vi "fast scanner v1.2.vi"() -> ()   [LabVIEW 2015]
uses:
  libs/Controls/outofrange.ctl
  libs/Controls/loopclock.ctl
  libs/Controls/fast scanner.ctl
  <vilib>/Utility/file.llb/Write Delimited Spreadsheet (DBL).vi
  <vilib>/Utility/file.llb/Write Delimited Spreadsheet (I64).vi
  Zaber A Series/Zaber A Series.lvlib
panel:
  out "DPP Configuration":T1={"reset_recovery_time"=300, "edge_peaking_time"=5, "flat_top"=5, "peaking_time"=25, "gain"=1.0, "max_risetime"=35.0, "fast_filter_thr"=100, "zero_peak_freq"=5.0, "inverted_input"=0, "base_offset"=0, "reset_threshold"=1000, "overflow_recovery"=0, "tail_coefficient"=0.0, "energy_filter_thr"=25, "energy_baseline_thr"=25, "max_peaking_time"=0, "edge_flat_top"=1, "time_constant"=0.0, "baseline_samples"=64, "other_param"=0}
  in  "Data folder path":path=path "d:/Users/XRF/Desktop/Scan DATA"
  out "DANTE loaded":bool
  out "IP added":bool
  out "Library Initialized":bool
  out "DANTE configured":bool
  out "Enum":T2=enum."MoveToStartPoint"
  out "scan mode":bool
  out "Port":refnum<visa-resource-name>
  out "MotorsReady":bool
  out "Speed 2":T3 scale=0.0..30.0
  in  "Tab Control":T4(tab)
  in  "StopMotion":bool
  in  "GoToZ":bool
  in  "GoToY":bool
  in  "GoToX":bool
  in  "GoTo Z [mm]":dbl format="%#.8g"
  in  "GoTo Y [mm]":dbl format="%#.8g"
  in  "GoTo X [mm]":dbl format="%#.8g"
  in  "Reduced Speed":bool
  in  "Speed Z [mm/s]":dbl(slide) caption="Z Speed\n[mm/s]" min=0.5 max=10.0 step=0.5 scale=0.5..10.0
  in  "XY Speed\n[mm/s]":dbl(slide)=1.0 min=1.0 max=75.0 step=1.0 scale=1.0..75.0
  in  "Away":bool
  in  "Closer":bool
  in  "Right":bool
  in  "Left":bool
  in  "Down":bool
  in  "Up":bool
  out "X [mm]":dbl format="%#.8g"
  out "Y [mm]":dbl format="%#.8g"
  out "Z [mm]":dbl format="%#.3g"
  out "Assignment":cluster{"Microstep Size":dbl, "Device":string}[](array[cluster])
  in  "Acceleration [mm/s^2]":dbl=1.0 min=1.0 max=488.0
  out "SpectraPlot":dbl[](graph) caption="Waveform Graph"
  in  "APPEARANCE_CursorVis":bool
  in  "APPEARANCE_Log/Lin":bool=TRUE
  out "stats out":T5
  out "identifier out":string
  in  "IP Address":string="10.96.0.110"
  out "Progress":u32 caption="%" min=1 step=1
  in  "Preset Time [s]":dbl=1.0 min=0.2 step=0.1
  out "Elapsed Time":dbl caption="Elapsed Time [s]" format="%#_4g"
  in  "MEASUREMENT_Start":bool
  in  "INIT DANTE":bool
  in  "Close DANTE":bool
  out "ROI Begin":u32 caption="ROI begin channel"
  out "ROI End":u32 caption="ROI end channel"
  in  "Config. file path":path=path "Configuration files/DefaultParameters.xml"
  in  "And dist [mm]":dbl=1.0 caption="Single line measurement time:" min=0.0 step=0.1
  in  "X velocity [mm/s]":dbl=50.0 min=0.0 step=0.1
  out "Total scan time [s]":dbl=1.0 min=0.0 step=0.1
  out "Total line time [s]":dbl=1.0 min=0.0 step=0.1
  out "Acq time [s]":dbl=1.0 min=0.0 step=0.1
  in  "AcqStartDelay":dbl caption="Acq start delay [ms]"
  in  "Abort scan":bool
  out "Acc time [s]":dbl=1.0 min=0.0 step=0.1
  out "Acc dist [mm]":dbl=1.0 caption="Single line measurement time:" min=0.0 step=0.1
  in  "X accel":dbl caption="X acceleration [mm/s^2]"
  out "Line #":i32=1 caption="/" min=0 step=1
  out "X scan velocity [mm/s]":dbl=1.0 min=0.0 step=0.1
  in  "QUICKSCAN_Start":bool
  out "Y error":T6
  out "X error":T6
  out "total # of points":i32=1 min=0 step=1
  out "Y steps":i32=1 min=1 step=1
  out "X steps":i32=1 min=1 step=1
  in  "step Y [mm]":dbl=1.0 min=0.0 step=0.1
  in  "Y end [mm]":dbl=1.0
  in  "Y start [mm]":dbl
  in  "step X [mm]":dbl=1.0 min=0.0 step=0.1
  in  "X end [mm]":dbl=1.0
  in  "X start [mm]":dbl
  in  "PresetVal":u32 caption="Time per pixel [ms]"
  out "X speed error":T6
  out "total line #":i32=1 caption="/" min=0 step=1
  out "Return movement time [s]":dbl=1.0 min=0.0 step=0.1
  out "ROI map":u32[][](graph)
  out "Sum spectra per line":u32[](graph)
  out "Spectra":u16[][](graph)
  out "scan timing [ms]":dbl[][](array[numeric])
  out "Y positions array":dbl[](array[numeric])
  out "X start position":dbl
  out "X end position":dbl
  in  "Precision [mm]":dbl=0.1
  out "ZaberError":errorcluster
  out "Loop Speed [1/s]":dbl caption="Elapsed Time [s]" format="%#_2f"
  # "waiting \ntill stage \nreaches \nproper speed"
  # "sending \nmovement \ncommand"
  # "waiting till \nstage stops \n(breaking)"
  # "aquisition"
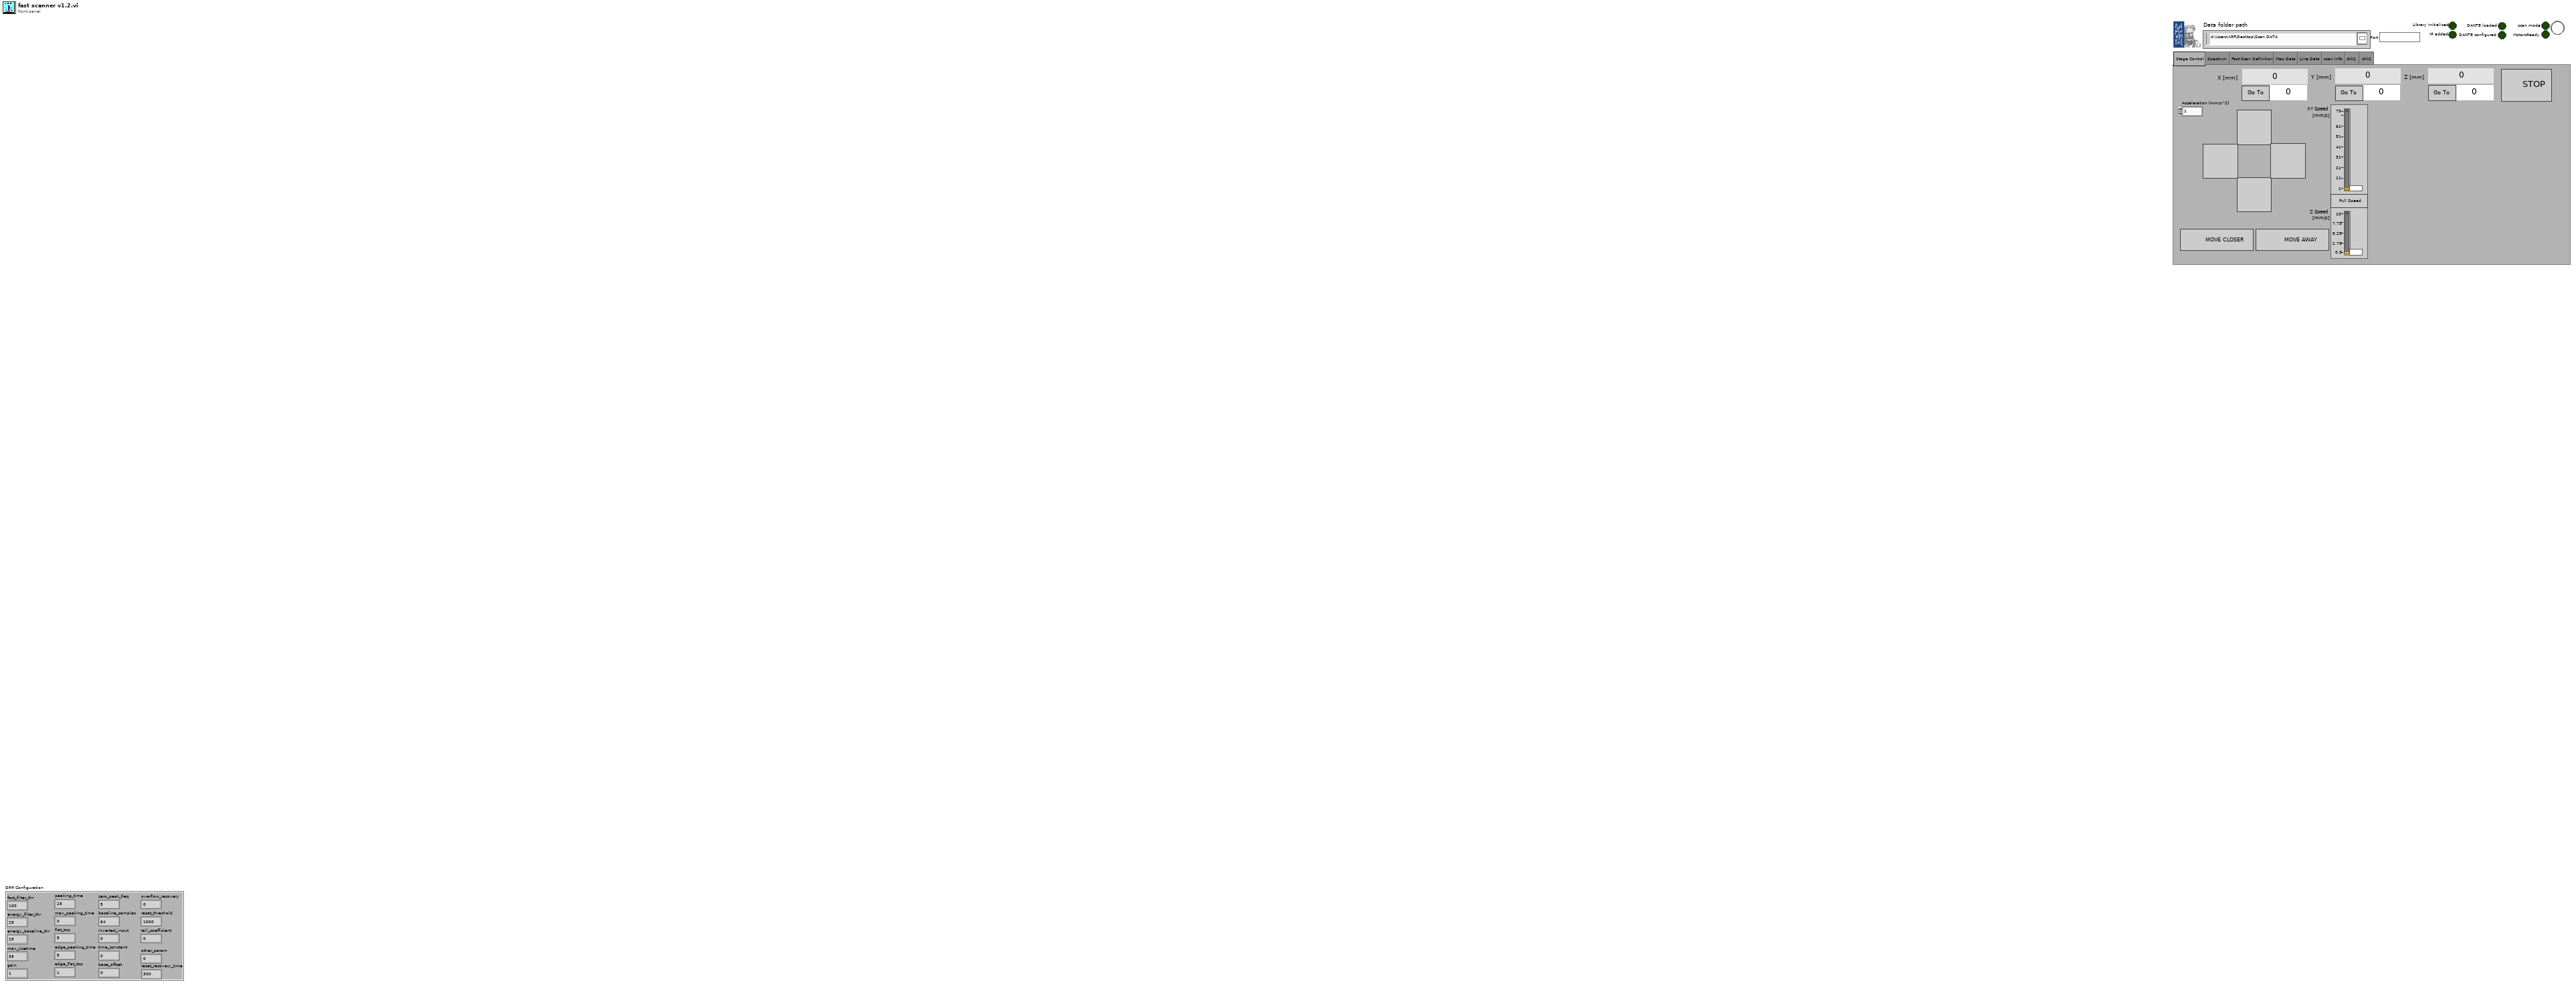
[diagram p1: front panel]
types:
  T1 = cluster{"reset_recovery_time":u32, "edge_peaking_time":u32, "flat_top":u32, "peaking_time":u32, "gain":dbl, "max_risetime":dbl, "fast_filter_thr":u32, "zero_peak_freq":dbl, "inverted_input":u8, "base_offset":u32, "reset_threshold":u32, "overflow_recovery":u32, "tail_coefficient":dbl, "energy_filter_thr":u32, "energy_baseline_thr":u32, "max_peaking_time":u32, "edge_flat_top":u32, "time_constant":dbl, "baseline_samples":u32, "other_param":u32}
  T2 = typedef "fast scanner.ctl" = enum16{"Initialisation", "IDLE", "Acquire", "PrepareMap", "MoveToStartPoint", "AcquireLine", "Close"}
  T3 = typedef "loopclock.ctl" = dbl
  T4 = enum32{"Stage Control", "Spectrum", "Fast Scan Definition", "Map Data", "Line Data", "scan info", "chk1", "chk2"}
  T5 = cluster{u64, u64, dbl, dbl, u32, u32, u32, u32, u32, u32, u32, u32, u32, u32, u32}
  T6 = typedef "outofrange.ctl" = bool
  T7 = cluster{"X min":dbl, "X max":dbl, "Y min":dbl, "Y max":dbl, "Z min":dbl, "Z max":dbl}
  T8 = enum32{"Size Tabs To Contents", "Size All Tabs to Largest Tab", "Fixed Tab Size"}
  T9 = enum8{"Enabled", "Disabled", "Disabled and Grayed Out"}
  T10 = typedef "ConfigurationDPP.ctl" = cluster{"reset_recovery_time":u32, "edge_peaking_time":u32, "flat_top":u32, "peaking_time":u32, "gain":dbl, "max_risetime":dbl, "fast_filter_thr":u32, "zero_peak_freq":dbl, "inverted_input":u8, "base_offset":u32, "reset_threshold":u32, "overflow_recovery":u32, "tail_coefficient":dbl, "energy_filter_thr":u32, "energy_baseline_thr":u32, "max_peaking_time":u32, "edge_flat_top":u32, "time_constant":dbl, "baseline_samples":u32, "other_param":u32}
  T11 = typedef "LVMinMaxIncTypeDef.ctl" = cluster{"Minimum":dbl, "Maximum":dbl, "Increment":dbl}
  T12 = typedef "LVRangeTypeDef.ctl" = cluster{"Minimum":dbl, "Maximum":dbl, "Increment":dbl, "Minor Increment":dbl, "Start":dbl}
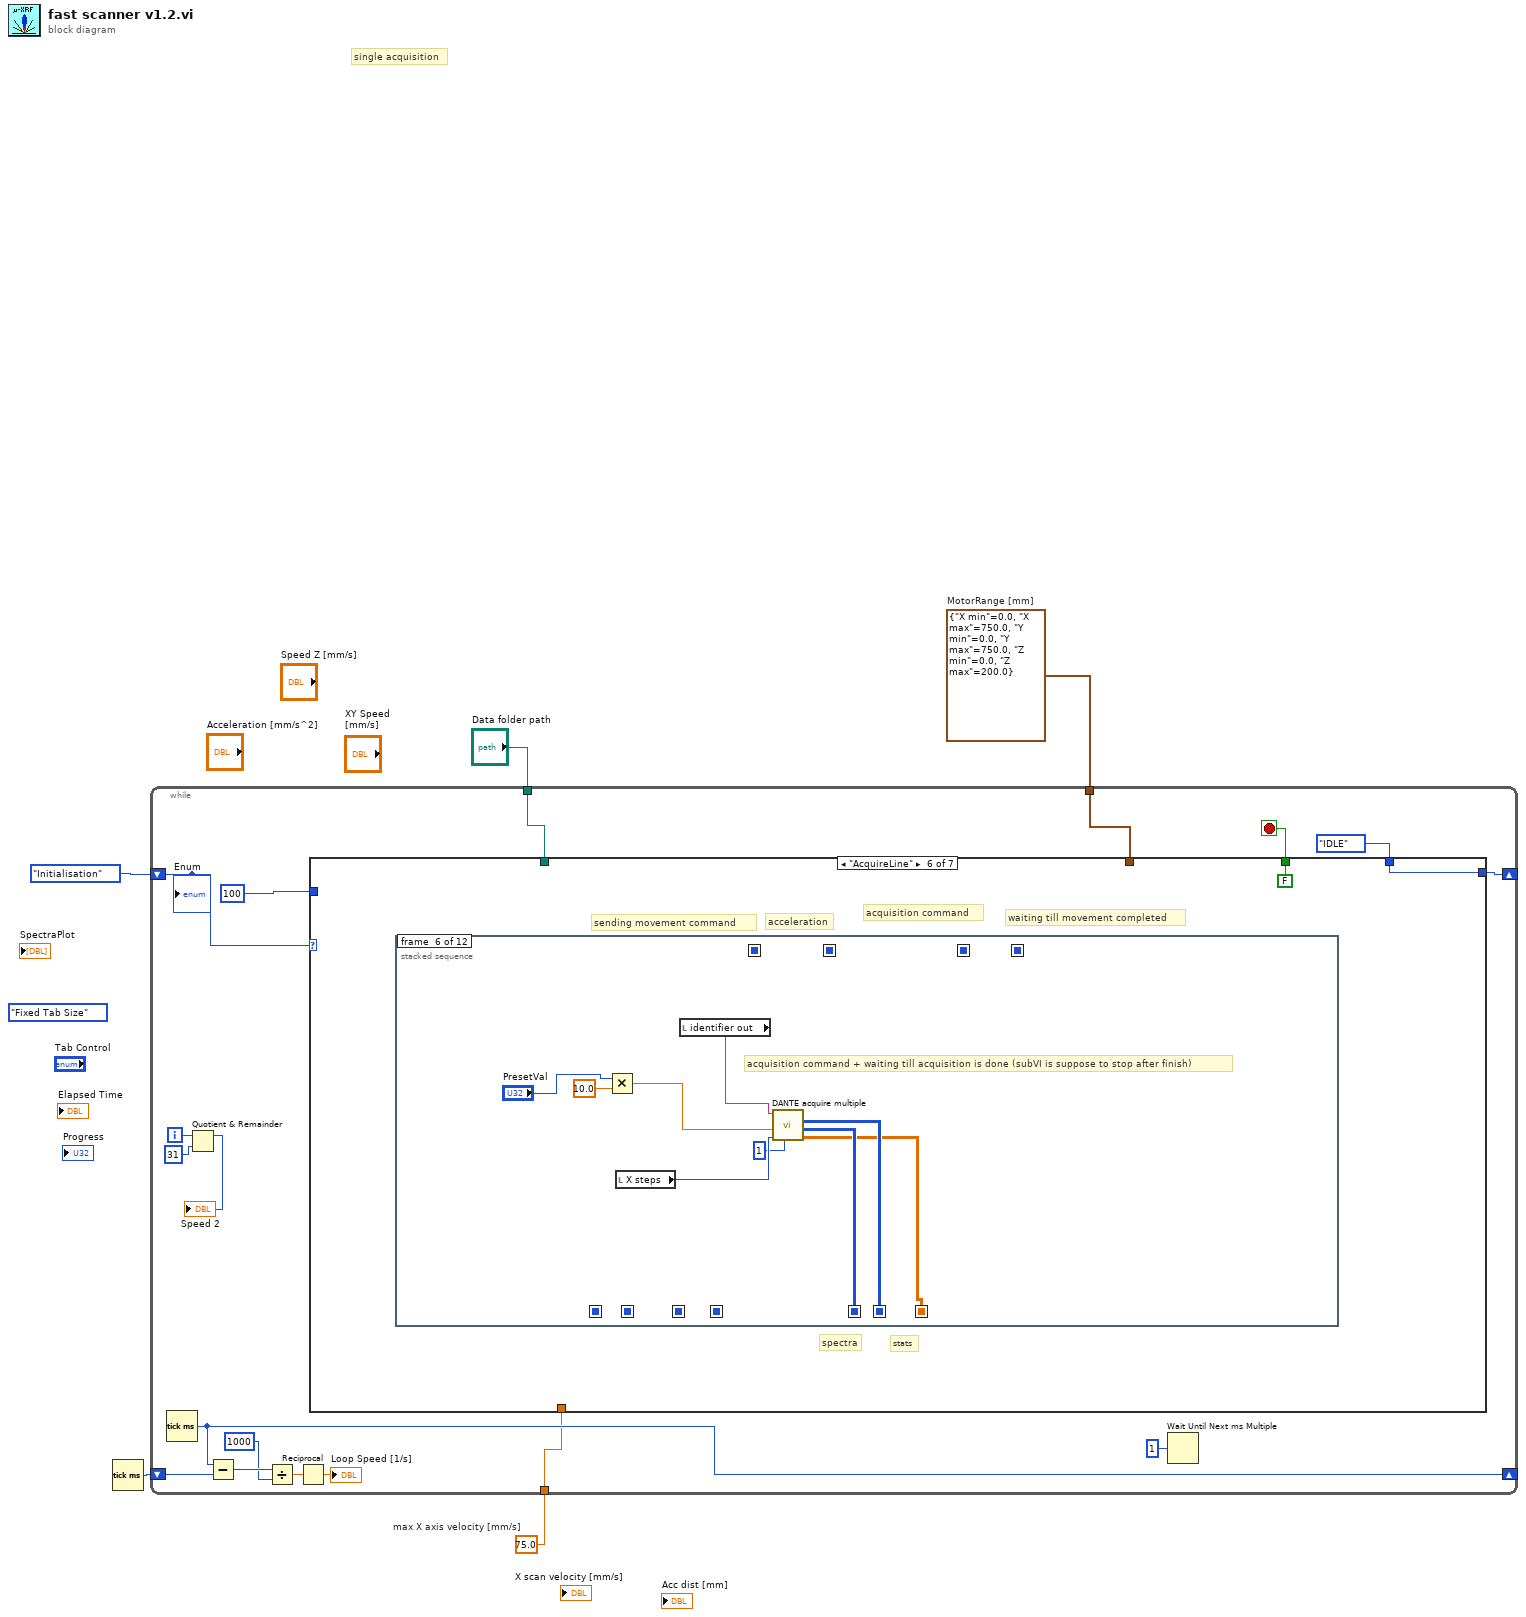
[diagram p0: block diagram]
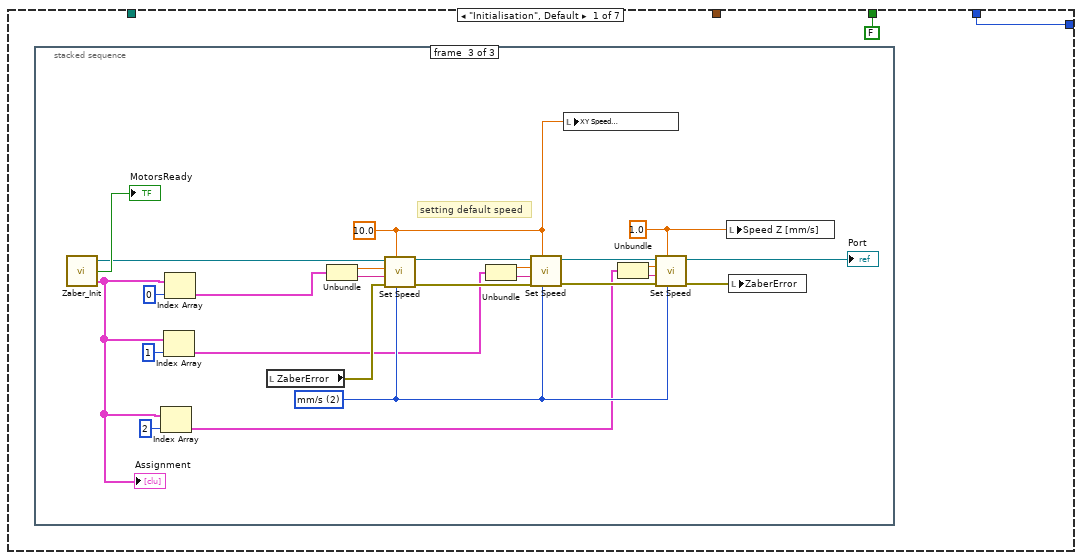
[diagram p2: hidden frame]
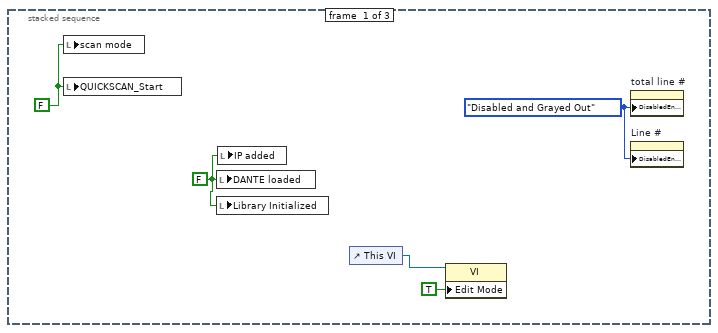
[diagram p3: hidden frame]
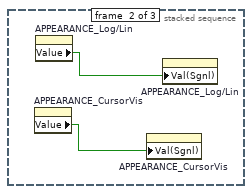
[diagram p4: hidden frame]
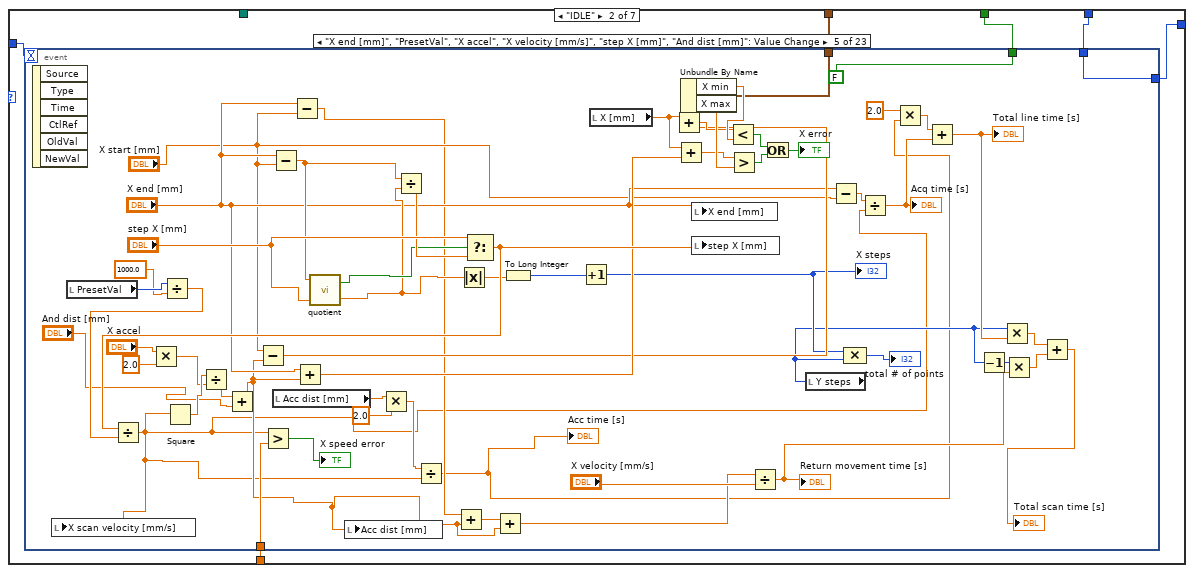
[diagram p5: hidden frame]
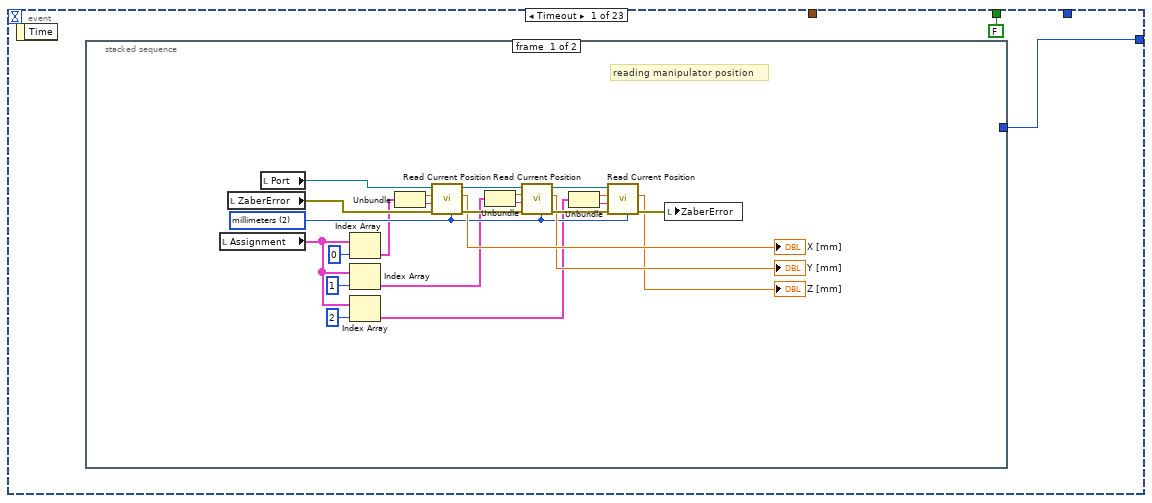
[diagram p6: hidden frame]
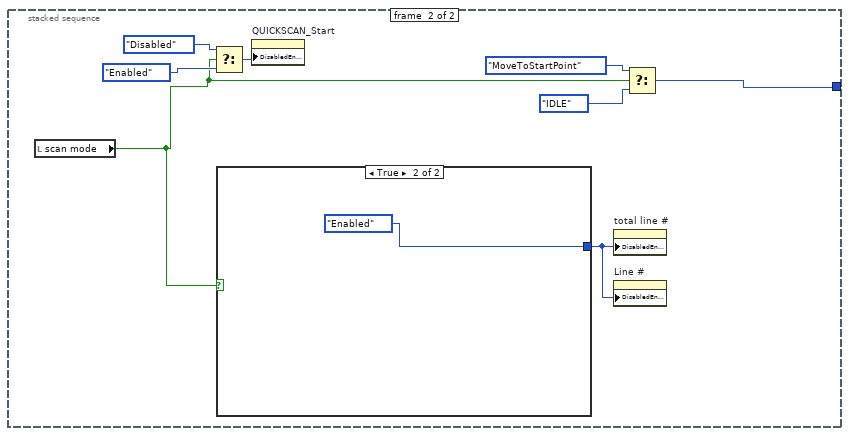
[diagram p7: hidden frame]
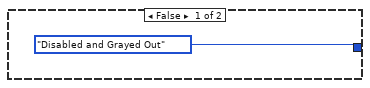
[diagram p8: hidden frame]
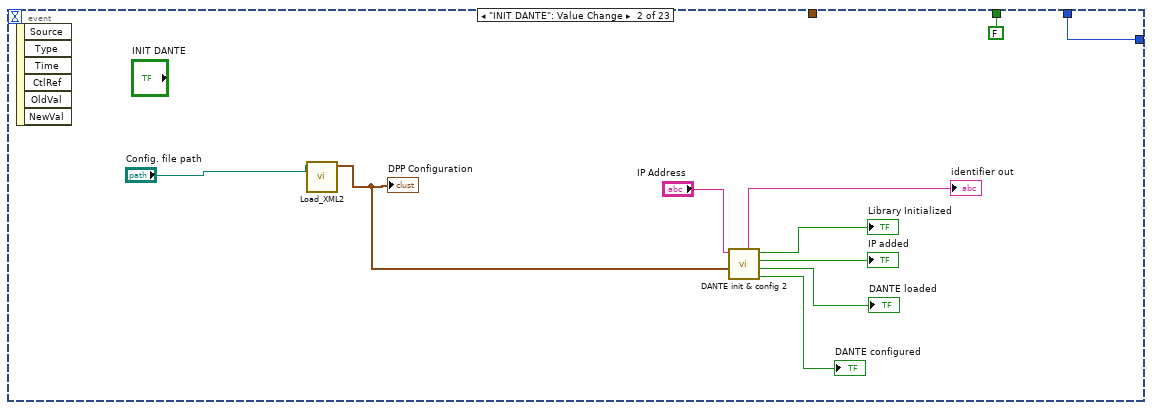
[diagram p9: hidden frame]
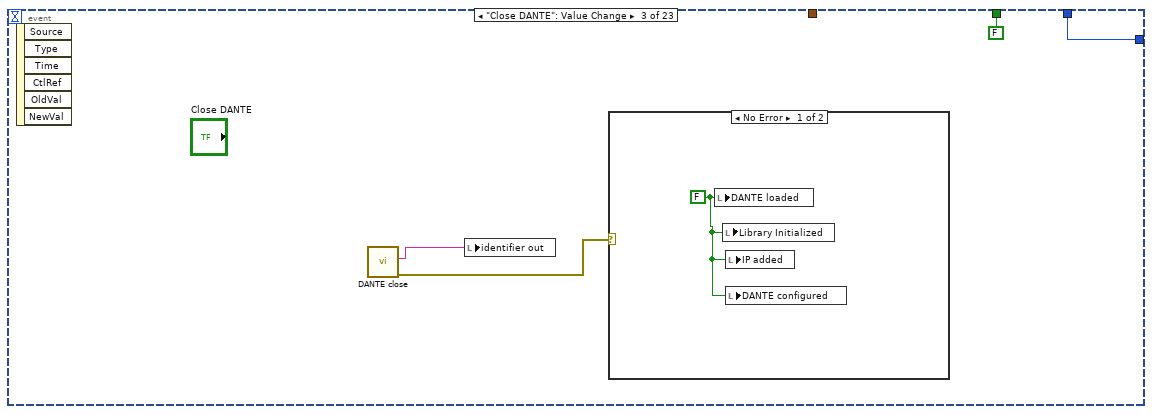
[diagram p10: hidden frame]
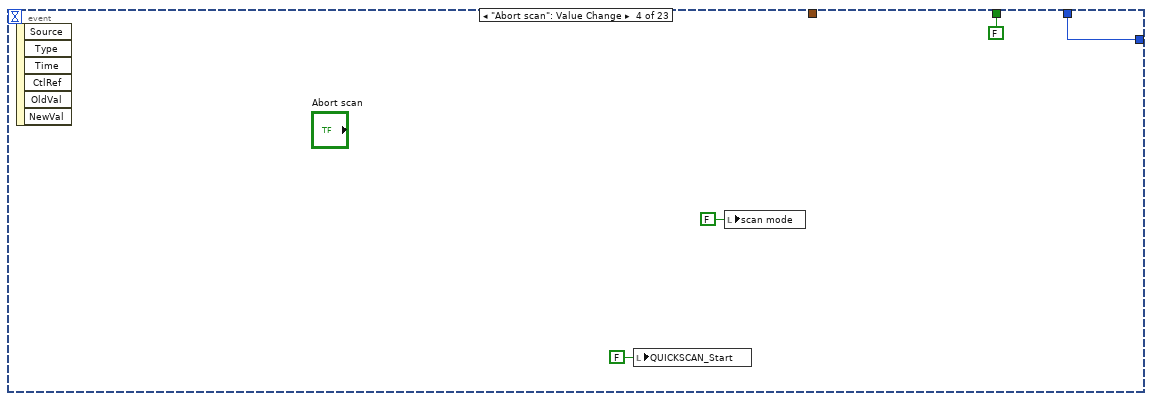
[diagram p12: hidden frame]
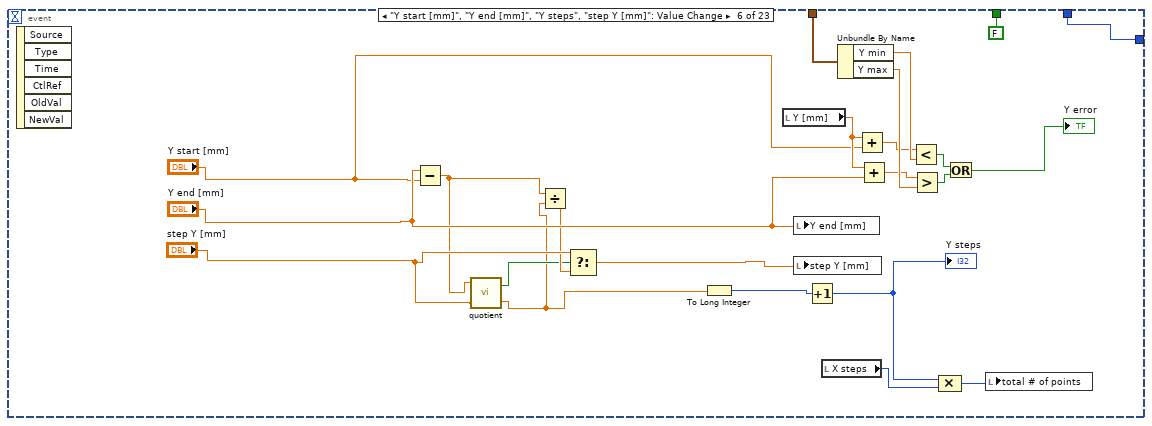
[diagram p13: hidden frame]
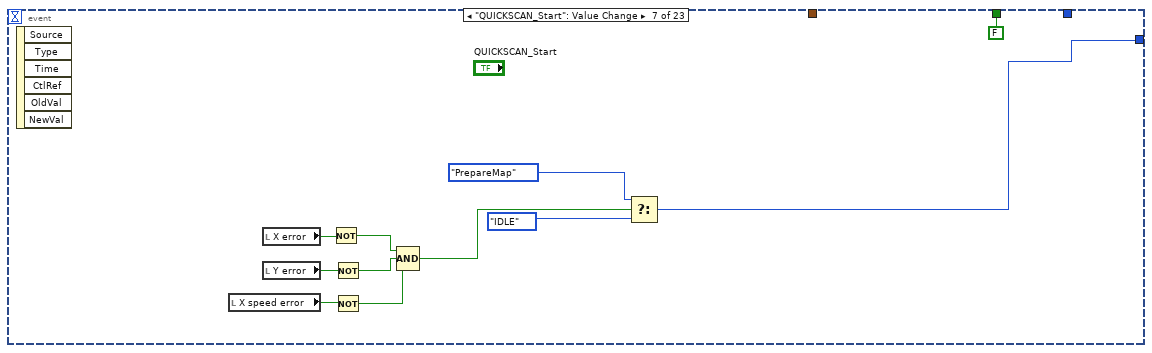
[diagram p14: hidden frame]
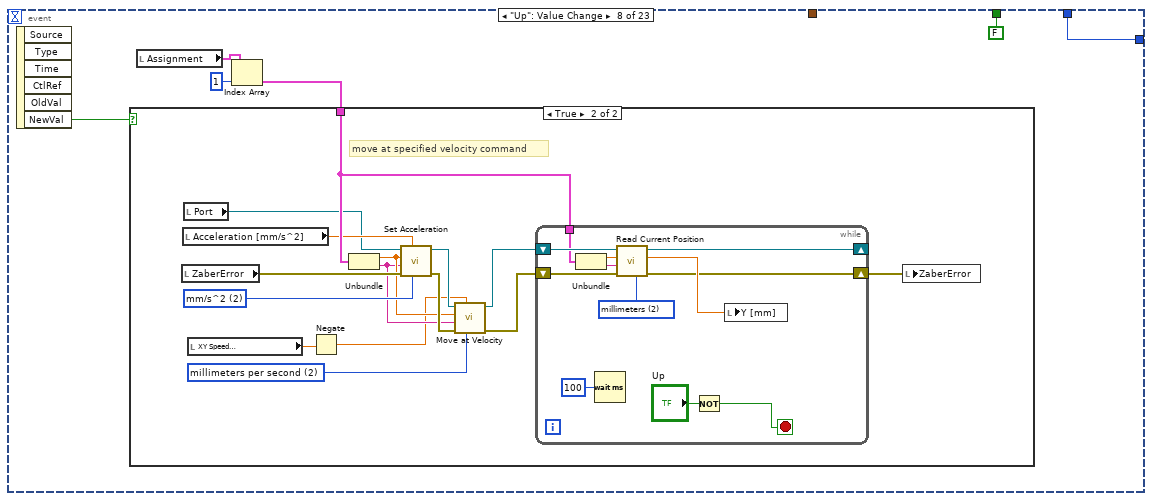
[diagram p15: hidden frame]
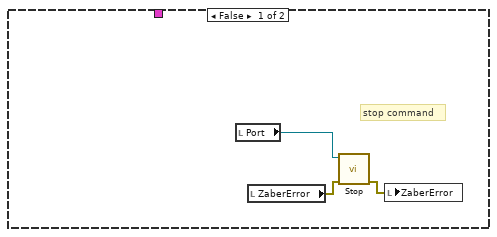
[diagram p16: hidden frame]
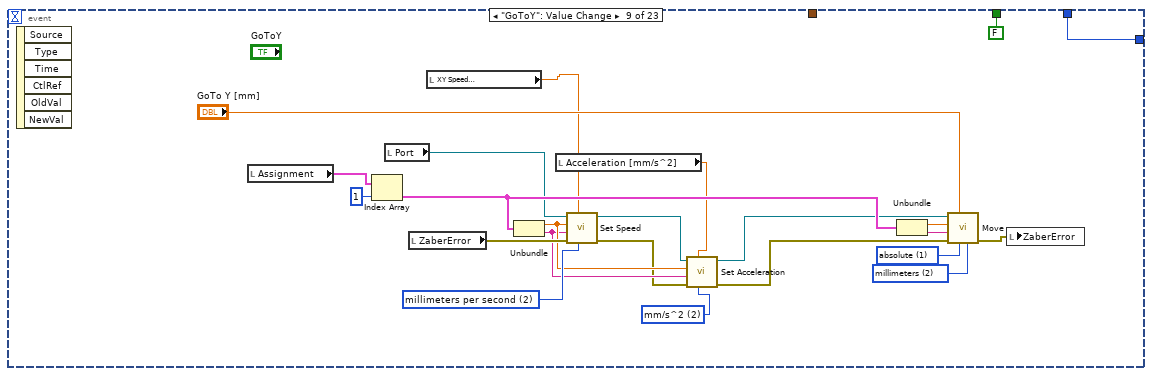
[diagram p17: hidden frame]
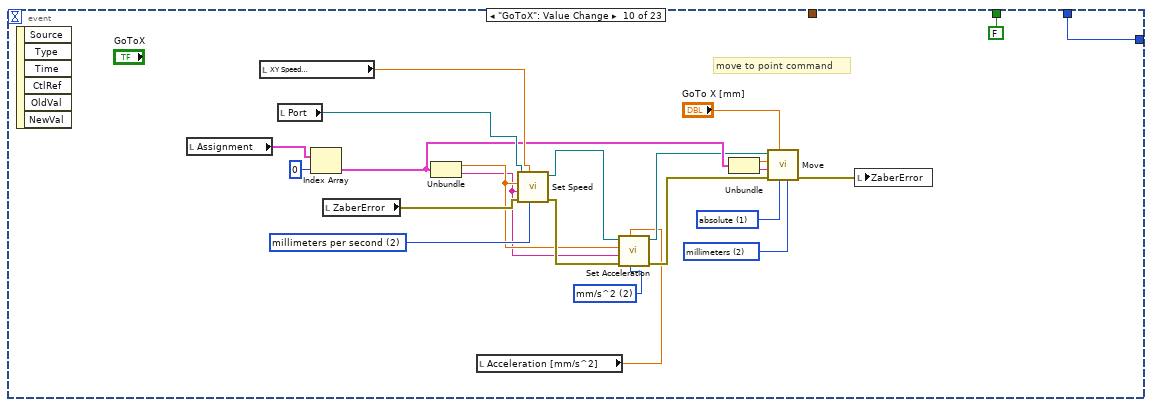
[diagram p18: hidden frame]
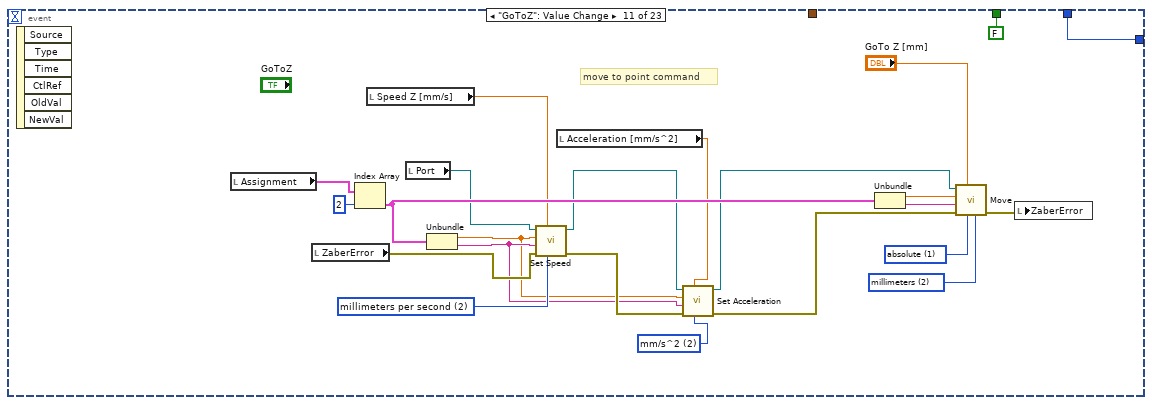
[diagram p19: hidden frame]
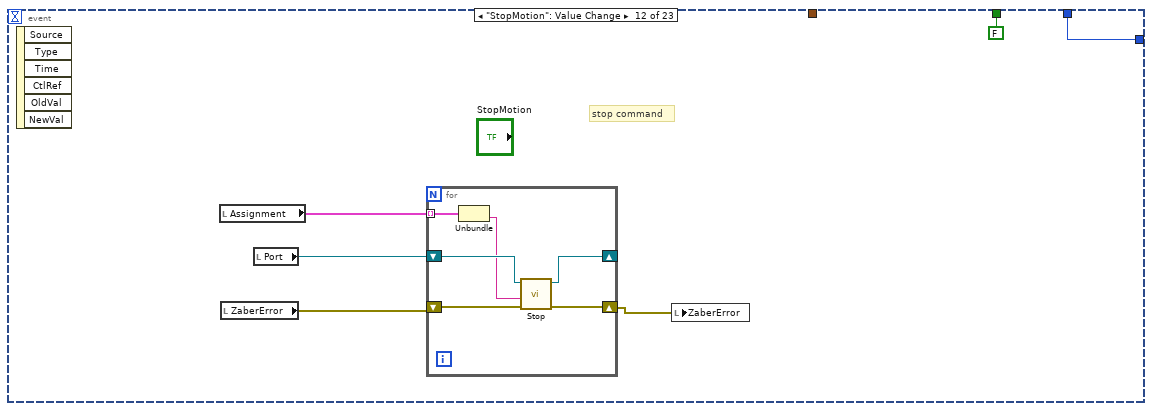
[diagram p20: hidden frame]
diagram:
  w2 = 75.0  # max X axis velocity [mm/s]
  w4 = T7 {"X min"=0.0, "X max"=750.0, "Y min"=0.0, "Y max"=750.0, "Z min"=0.0, "Z max"=200.0}  # MotorRange [mm]
  (unwired) T8."Fixed Tab Size" ("Tab Size")
  # "single acquisition"
  n1 = Tick Count (ms)() -> (millisecond timer value=w5:u32)
  n2 = while {
    shift-right: [w12] -> _
    shift-left: fast_scanner."Initialisation" ("Enum") -> [w8]
    shift-right: [w19] -> _
    shift-left: w5 -> [w23]
    tunnel: w4 -> [w9]
    tunnel: w2 -> [w7]
    tunnel: "Data folder path" -> [w6]
    i -> [w18]
    stop <- w11 stop-if-true
    n3 = Tick Count (ms)() -> (millisecond timer value=w19:u32)
    n4 = Quotient & Remainder(x=w18, y=31) -> (x-y*floor(x/y)=→"Speed 2":i32)  [unwired: 1 out]
    n5 = Subtract(x=w19, y=w23) -> (x-y=w21:u32)
    n6 = Divide(x=w21, y=u32 1000) -> (x/y=w22:dbl)
    n7 = Reciprocal(x=w22) -> (1/x=→"Loop Speed [1/s]":dbl)
    n8 = case shown="\"AcquireLine\"" w8 {
      tunnel: 100 ("LoopTimer [ms]") -> [_ w59 _ _ _ _ _]
      tunnel: [w25 w61 fast_scanner."IDLE" ("Enum") w582 fast_scanner."AcquireLine" ("Enum") w692 fast_scanner."Close" ("Enum")] -> w12
      tunnel: [FALSE ("VI stop") w60 FALSE ("VI stop") FALSE ("VI stop") FALSE ("VI stop") FALSE ("VI stop") TRUE ("VI stop")] -> w11
      tunnel: fast_scanner."IDLE" ("Enum") -> [w25 w63 _ w582 _ w692 _]
      tunnel: w9 -> [_ w62 _ _ _ _ _]
      tunnel: w7 -> [_ w58 _ _ _ _ _]
      tunnel: w6 -> [_ _ _ _ _ _ _]
      frame "Initialisation", Default {
        n9 = stacked-sequence {
          frame #0 {
            w26 = FALSE ("DANTE loaded")
            w27 = T9."Disabled and Grayed Out" ("Disabled")
            w28 = FALSE ("batch mode")
            n10 = local write "scan mode"(w28) -> ()
            n11 = local write "QUICKSCAN_Start"(w28) -> ()
            n12 = local write "DANTE loaded"(w26) -> ()
            n13 = local write "Library Initialized"(w26) -> ()
            n14 = local write "IP added"(w26) -> ()
            n15 = control-ref of="This VI"() -> (w29:refnum<vi>)
            n16 = property class="VI"(reference=w29, "Edit Mode"=TRUE ("Edit Mode On Open")) -> ()  [unwired: 1 in, 2 out]
            n17 = property on="total line #" class="DigNum (strict)"("DisabledEnum"=w27) -> ()  [unwired: 2 in, 2 out]
            n18 = property on="Line #" class="DigNum (strict)"("DisabledEnum"=w27) -> ()  [unwired: 2 in, 2 out]
          }
          frame #1 {
            n19 = property on="APPEARANCE_CursorVis" class="Bool (strict)"() -> ("Value"=w31:bool)  [unwired: 2 in, 2 out]
            n20 = property on="APPEARANCE_Log/Lin" class="Bool (strict)"() -> ("Value"=w32:bool)  [unwired: 2 in, 2 out]
            n21 = property on="APPEARANCE_CursorVis" class="Bool (strict)"("Val(Sgnl)"=w31) -> ()  [unwired: 2 in, 2 out]
            n22 = property on="APPEARANCE_Log/Lin" class="Bool (strict)"("Val(Sgnl)"=w32) -> ()  [unwired: 2 in, 2 out]
          }
          frame #2 {
            w42 = 1.0 ("New Speed")
            w43 = 10.0 ("New Speed")
            w46 = u16 2 items=["device units", "microns/s", "mm/s", "inches/s", "degrees/s"] ("Units (0: data)")
            # "setting default speed"
            n23 = call "Zaber_Init.vi"() -> ("Assignment"=w47:cluster{"Microstep Size":dbl, "Device":string}[], "Axes Ass"=→"MotorsReady":bool, "VISA resource name out"=w55:refnum<visa-resource-name>)
            "Assignment" <- w47
            n24 = Index Array(array=w47, index=2) -> (element=w34:cluster{"Microstep Size":dbl, "Device":string})
            n25 = Index Array(array=w47, index=1) -> (element=w36:cluster{"Microstep Size":dbl, "Device":string})
            n26 = Index Array(array=w47, index=0) -> (element=w41:cluster{"Microstep Size":dbl, "Device":string})
            n27 = local read "ZaberError"() -> (w56:errorcluster)
            n28 = Unbundle(w41) -> ("Microstep Size"=w40:dbl, "Device"=w39:string)
            n29 = call "Set Speed.vi"("Units (0: data)"=w46, "New Speed"=w43, "error in (no error)"=w56, "Device and Axis"=w39, "Microstep Size (0)"=w40, "VISA resource name"=w55) -> ("error out"=w52:errorcluster, "VISA resource name out"=w51:refnum<visa-resource-name>)  [unwired: 4 in]
            n30 = Unbundle(w36) -> ("Microstep Size"=w37:dbl, "Device"=w38:string)
            n31 = call "Set Speed.vi"("Units (0: data)"=w46, "New Speed"=w43, "error in (no error)"=w52, "Device and Axis"=w38, "Microstep Size (0)"=w37, "VISA resource name"=w51) -> ("error out"=w49:errorcluster, "VISA resource name out"=w50:refnum<visa-resource-name>)  [unwired: 4 in]
            n32 = local write "XY Speed\n[mm/s]"(w43) -> ()
            n33 = Unbundle(w34) -> ("Microstep Size"=w35:dbl, "Device"=w33:string)
            n34 = call "Set Speed.vi"("Units (0: data)"=w46, "New Speed"=w42, "error in (no error)"=w49, "Device and Axis"=w33, "Microstep Size (0)"=w35, "VISA resource name"=w50) -> ("error out"=w45:errorcluster, "VISA resource name out"=→"Port":refnum<visa-resource-name>)  [unwired: 4 in]
            n35 = local write "Speed Z [mm/s]"(w42) -> ()
            n36 = local write "ZaberError"(w45) -> ()
          }
        }
      }
      frame "IDLE" {
        n37 = event shown="[4] \"X end [mm]\", \"PresetVal\", \"X accel\", \"X velocity [mm/s]\", \"step X [mm]\", \"And dist [mm]\": Value Change" {
          selector: _ -> [_ _ _ _ _ _ _ _ _ _ _ _ _ _ _ _ _ _ _ _ _ _ _]
          dyn-events: _ -> [_ _ _ _ _ _ _ _ _ _ _ _ _ _ _ _ _ _ _ _ _ _ _]
          timeout: w59 -> [_ _ _ _ _ _ _ _ _ _ _ _ _ _ _ _ _ _ _ _ _ _ _]
          tunnel: [FALSE ("VI stop") FALSE ("VI stop") FALSE ("VI stop") FALSE ("VI stop") FALSE ("VI stop") FALSE ("VI stop") FALSE ("VI stop") FALSE ("VI stop") FALSE ("VI stop") FALSE ("VI stop") FALSE ("VI stop") FALSE ("VI stop") FALSE ("VI stop") FALSE ("VI stop") FALSE ("VI stop") FALSE ("VI stop") FALSE ("VI stop") FALSE ("VI stop") TRUE ("VI stop") FALSE ("VI stop") FALSE ("VI stop") FALSE ("VI stop") FALSE ("VI stop")] -> w60
          tunnel: [w64 w109 w113 w117 w175 w196 w199 w213 w267 w290 w313 w320 w331 w366 w401 w437 w472 w516 w533 fast_scanner."Acquire" ("Enum") w551 w556 w560] -> w61
          tunnel: w63 -> [_ w109 w113 w117 w175 w196 _ w213 w267 w290 w313 w320 w331 w366 w401 w437 w472 w516 _ _ w551 w556 w560]
          tunnel: w62 -> [_ _ _ _ w163 w182 _ _ _ _ _ _ _ _ _ _ _ _ _ _ _ _ _]
          tunnel: w58 -> [_ _ _ _ w152 _ _ _ _ _ _ _ _ _ _ _ _ _ _ _ _ _ _]
          event Timeout {
            n38 = event-data() -> ()  [unwired: 1 in, 1 out]
            n39 = stacked-sequence {
              tunnel: [_ w97] -> w64
              frame #0 {
                w76 = u16 2 items=["microsteps", "microns", "millimeters", "inches"] ("Units (0: microsteps)")
                # "reading manipulator position"
                n40 = local read "Assignment"() -> (w75:cluster{"Microstep Size":dbl, "Device":string}[])
                n41 = local read "ZaberError"() -> (w88:errorcluster)
                n42 = local read "Port"() -> (w89:refnum<visa-resource-name>)
                n43 = Index Array(array=w75, index=0) -> (element=w74:cluster{"Microstep Size":dbl, "Device":string})
                n44 = Index Array(array=w75, index=1) -> (element=w70:cluster{"Microstep Size":dbl, "Device":string})
                n45 = Index Array(array=w75, index=2) -> (element=w66:cluster{"Microstep Size":dbl, "Device":string})
                n46 = Unbundle(w74) -> ("Microstep Size"=w73:dbl, "Device"=w72:string)
                n47 = call "Read Current Position.vi"("Units (0: microsteps)"=w76, "error in (no error)"=w88, "Device and Axis"=w72, "Microstep Size (0)"=w73, "VISA resource name"=w89) -> ("error out"=w87:errorcluster, "Position"=→"X [mm]":dbl, "VISA resource name out"=w86:refnum<visa-resource-name>)  [unwired: 4 in]
                n48 = Unbundle(w70) -> ("Microstep Size"=w71:dbl, "Device"=w69:string)
                n49 = call "Read Current Position.vi"("Units (0: microsteps)"=w76, "error in (no error)"=w87, "Device and Axis"=w69, "Microstep Size (0)"=w71, "VISA resource name"=w86) -> ("error out"=w85:errorcluster, "Position"=→"Y [mm]":dbl, "VISA resource name out"=w84:refnum<visa-resource-name>)  [unwired: 4 in]
                n50 = Unbundle(w66) -> ("Microstep Size"=w68:dbl, "Device"=w67:string)
                n51 = call "Read Current Position.vi"("Units (0: microsteps)"=w76, "error in (no error)"=w85, "Device and Axis"=w67, "Microstep Size (0)"=w68, "VISA resource name"=w84) -> ("error out"=w83:errorcluster, "Position"=→"Z [mm]":dbl)  [unwired: 4 in, 1 out]
                n52 = local write "ZaberError"(w83) -> ()
              }
              frame #1 {
                n53 = local read "scan mode"() -> (w90:bool)
                n54 = Select(t=T9."Disabled" ("Disabled"), s=w90, f=T9."Enabled" ("Disabled")) -> (s? t:f=w94:T9)
                n55 = case shown="True" w90 {
                  tunnel: [T9."Disabled and Grayed Out" ("Disabled") T9."Enabled" ("Disabled")] -> w91
                  frame False {
                  }
                  frame True {
                  }
                }
                n56 = property on="QUICKSCAN_Start" class="Bool (strict)"("DisabledEnum"=w94) -> ()  [unwired: 2 in, 2 out]
                n57 = property on="total line #" class="DigNum (strict)"("DisabledEnum"=w91) -> ()  [unwired: 2 in, 2 out]
                n58 = property on="Line #" class="DigNum (strict)"("DisabledEnum"=w91) -> ()  [unwired: 2 in, 2 out]
                n59 = Select(t=fast_scanner."MoveToStartPoint" ("Enum"), s=w90, f=fast_scanner."IDLE" ("Enum")) -> (s? t:f=w97:T2)
              }
            }
          }
          event "INIT DANTE": Value Change {
            n60 = event-data() -> ()  [unwired: 1 in, 6 out]
            n61 = call "Load_XML2.vi"("XML File Path 2"="Config. file path") -> ("DPP Configuration"=w100:T10)  [unwired: 10 in]
            "DPP Configuration" <- w100
            n62 = call "DANTE init & config 2.vi"("DPP Configuration"=w100, "IP Address"="IP Address") -> ("DANTE configured"=→"DANTE configured":bool, "DANTE loaded"=→"DANTE loaded":bool, "IP added"=→"IP added":bool, "Library Initialized"=→"Library Initialized":bool, "identifier out"=→"identifier out":string)  [unwired: 5 in]
          }
          event "Close DANTE": Value Change {
            n63 = event-data() -> ()  [unwired: 1 in, 6 out]
            n64 = call "DANTE close.vi"() -> ("error out"=w110:errorcluster, "identifier out"=w111:string)  [unwired: 9 in, 1 out]
            n65 = local write "identifier out"(w111) -> ()
            n66 = case shown="No Error" w110 {
              frame No Error {
                w114 = FALSE ("DANTE loaded")
                n67 = local write "DANTE loaded"(w114) -> ()
                n68 = local write "Library Initialized"(w114) -> ()
                n69 = local write "IP added"(w114) -> ()
                n70 = local write "DANTE configured"(w114) -> ()
              }
              frame Error {
              }
            }
          }
          event "Abort scan": Value Change {
            n71 = event-data() -> ()  [unwired: 1 in, 6 out]
            n72 = local write "QUICKSCAN_Start"(FALSE ("QUICKSCAN_Start")) -> ()
            n73 = local write "scan mode"(FALSE ("scan mode")) -> ()
          }
          event "X end [mm]", "PresetVal", "X accel", "X velocity [mm/s]", "step X [mm]", "And dist [mm]": Value Change {
            n74 = event-data() -> ()  [unwired: 1 in, 6 out]
            n75 = local read "PresetVal"() -> (w159:u32)
            n76 = Multiply(x="X accel", y=2.0) -> (x*y=w154:dbl)
            n77 = Divide(x=w159, y=1000.0 ("x")) -> (x/y=w157:dbl)
            n78 = Subtract(x="X end [mm]", y="X start [mm]") -> (x-y=w146:dbl)
            n79 = local read "Acc dist [mm]"() -> (w124:dbl)
            n80 = Subtract(x="X end [mm]", y="X start [mm]") -> (x-y=w129:dbl)
            n81 = call "quotient.vi"("Y"="step X [mm]", "X"=w146) -> ("s? t:f"=w144:dbl, "x = y?"=w145:bool)  [unwired: 1 in]
            n82 = Multiply(x=w124, y=2.0) -> (x*y=w122:dbl)
            n83 = Divide(x=w146, y=w144) -> (x/y=w148:dbl)
            n84 = Absolute Value(x=w144) -> (abs(x)=w147:dbl)
            n85 = Select(t="step X [mm]", s=w145, f=w148) -> (s? t:f=w161:dbl)
            n86 = Divide(x=w161, y=w157) -> (x/y=w120:dbl)
            n87 = local write "X scan velocity [mm/s]"(w120) -> ()
            n88 = Square(x=w120) -> (x^2=w156:dbl)
            n89 = Divide(x=w156, y=w154) -> (x/y=w126:dbl)
            n90 = Add(x=w126, y="And dist [mm]") -> (x+y=w125:dbl)
            n91 = Subtract(x="X start [mm]", y=w125) -> (x-y=w150:dbl)
            n92 = Greater?(x=w120, y=w152) -> (0:→"X speed error":bool)
            n93 = Add(x="X end [mm]", y=w125) -> (x+y=w151:dbl)
            n94 = local write "Acc dist [mm]"(w125) -> ()
            n95 = Divide(x=w122, y=w120) -> (x/y=w119:dbl)
            "Acc time [s]" <- w119
            n96 = Add(x=w129, y=w125) -> (x+y=w128:dbl)
            n97 = Add(x=w128, y=w125) -> (x+y=w127:dbl)
            n98 = To Long Integer(number=w147) -> (32bit integer=w167:i32)
            n99 = Increment(x=w167) -> (x+1=w143:i32)
            "X steps" <- w143
            n100 = local read "X [mm]"() -> (w171:dbl)
            n101 = Add(x=w171, y=w150) -> (x+y=w166:dbl)
            n102 = Add(x=w171, y=w151) -> (x+y=w165:dbl)
            n103 = Unbundle By Name(w163) -> ("X min"=w172:dbl, "X max"=w170:dbl)
            n104 = local write "X end [mm]"("X end [mm]") -> ()
            n105 = local write "step X [mm]"(w161) -> ()
            n106 = Less?(x=w166, y=w172) -> (x < y?=w168:bool)
            n107 = Greater?(x=w165, y=w170) -> (0:w169:bool)
            n108 = Divide(x=w127, y="X velocity [mm/s]") -> (x/y=w135:dbl)
            "Return movement time [s]" <- w135
            n109 = Or(x=w168, y=w169) -> (x .or. y?=→"X error":bool)
            n110 = local read "Y steps"() -> (w136:i32)
            n111 = Subtract(x="X end [mm]", y="X start [mm]") -> (x-y=w142:dbl)
            n112 = Compound Arithmetic op=MULTIPLY(w143, w136) -> (→"total # of points":i32)
            n113 = Divide(x=w142, y=w120) -> (x/y=w141:dbl)
            "Acq time [s]" <- w141
            n114 = Multiply(x=2.0, y=w119) -> (x*y=w140:dbl)
            n115 = Add(x=w140, y=w141) -> (x+y=w138:dbl)
            "Total line time [s]" <- w138
            n116 = Decrement(x=w136) -> (x-1=w137:i32)
            n117 = Multiply(x=w136, y=w138) -> (x*y=w133:dbl)
            n118 = Multiply(x=w137, y=w135) -> (x*y=w134:dbl)
            n119 = Add(x=w133, y=w134) -> (x+y=→"Total scan time [s]":dbl)
          }
          event "Y start [mm]", "Y end [mm]", "Y steps", "step Y [mm]": Value Change {
            n120 = event-data() -> ()  [unwired: 1 in, 6 out]
            n121 = Subtract(x="Y end [mm]", y="Y start [mm]") -> (x-y=w179:dbl)
            n122 = call "quotient.vi"("Y"="step Y [mm]", "X"=w179) -> ("s? t:f"=w177:dbl, "x = y?"=w178:bool)  [unwired: 1 in]
            n123 = Divide(x=w179, y=w177) -> (x/y=w180:dbl)
            n124 = Select(t="step Y [mm]", s=w178, f=w180) -> (s? t:f=w183:dbl)
            n125 = To Long Integer(number=w177) -> (32bit integer=w194:i32)
            n126 = local read "Y [mm]"() -> (w192:dbl)
            n127 = local write "Y end [mm]"("Y end [mm]") -> ()
            n128 = local write "step Y [mm]"(w183) -> ()
            n129 = Increment(x=w194) -> (x+1=w176:i32)
            "Y steps" <- w176
            n130 = local read "X steps"() -> (w193:i32)
            n131 = Unbundle By Name(w182) -> ("Y min"=w188:dbl, "Y max"=w187:dbl)
            n132 = Add(x=w192, y="Y start [mm]") -> (x+y=w185:dbl)
            n133 = Add(x=w192, y="Y end [mm]") -> (x+y=w184:dbl)
            n134 = Less?(x=w185, y=w188) -> (x < y?=w190:bool)
            n135 = Greater?(x=w184, y=w187) -> (0:w191:bool)
            n136 = Compound Arithmetic op=MULTIPLY(w176, w193) -> (w181:i32)
            n137 = Or(x=w190, y=w191) -> (x .or. y?=→"Y error":bool)
            n138 = local write "total # of points"(w181) -> ()
          }
          event "QUICKSCAN_Start": Value Change {
            n139 = event-data() -> ()  [unwired: 1 in, 6 out]
            n140 = local read "X speed error"() -> (w205:T6)
            n141 = local read "X error"() -> (w203:T6)
            n142 = local read "Y error"() -> (w204:T6)
            n143 = Not(x=w203) -> (.not. x?=w206:T6)
            n144 = Not(x=w204) -> (.not. x?=w207:T6)
            n145 = Not(x=w205) -> (.not. x?=w208:T6)
            n146 = Compound Arithmetic op=AND(w206, w207, w208) -> (w202:T6)
            n147 = Select(t=fast_scanner."PrepareMap" ("Enum"), s=w202, f=fast_scanner."IDLE" ("Enum")) -> (s? t:f=w199:T2)
          }
          event "Up": Value Change {
            n148 = event-data() -> ("NewVal"=w215:bool)  [unwired: 1 in, 5 out]
            n149 = local read "Assignment"() -> (w210:cluster{"Microstep Size":dbl, "Device":string}[])
            n150 = Index Array(array=w210, index=1) -> (element=w211:cluster{"Microstep Size":dbl, "Device":string})
            n151 = case shown="True" w215 {
              tunnel: w211 -> [_ w232]
              frame False {
                # "stop command"
                n152 = local read "Port"() -> (w218:refnum<visa-resource-name>)
                n153 = local read "ZaberError"() -> (w217:errorcluster)
                n154 = call "Stop.vi"("error in (no error)"=w217, "VISA resource name"=w218) -> ("error out"=w216:errorcluster)  [unwired: 8 in, 1 out]
                n155 = local write "ZaberError"(w216) -> ()
              }
              frame True {
                w230 = u16 2 items=["device units", "microns/s^2", "mm/s^2", "inches/s^2", "degrees/s^2"] ("Units (0: data)")
                w220 = u16 2 items=["device speed units", "microns per second", "millimeters per second", "inches per second", "degrees per second"] ("Units (0: device speed units)")
                # "move at specified velocity command"
                n156 = local read "ZaberError"() -> (w228:errorcluster)
                n157 = local read "Acceleration [mm/s^2]"() -> (w229:dbl)
                n158 = local read "Port"() -> (w227:refnum<visa-resource-name>)
                n159 = local read "XY Speed\n[mm/s]"() -> (w231:dbl)
                n160 = Negate(x=w231) -> (-x=w219:dbl)
                n161 = Unbundle(w232) -> ("Microstep Size"=w224:dbl, "Device"=w223:string)
                n162 = call "Set Acceleration.vi"("Units (0: data)"=w230, "New Acceleration"=w229, "error in (no error)"=w228, "Device and Axis"=w223, "Microstep Size (0)"=w224, "VISA resource name"=w227) -> ("error out"=w226:errorcluster, "VISA resource name out"=w225:refnum<visa-resource-name>)  [unwired: 4 in]
                n163 = call "Move at Velocity.vi"("Units (0: device speed units)"=w220, "Velocity"=w219, "error in (no error)"=w226, "Device and Axis"=w223, "Microstep Size (0)"=w224, "VISA resource name"=w225) -> ("error out"=w221:errorcluster, "VISA resource name out"=w222:refnum<visa-resource-name>)  [unwired: 4 in]
                n164 = while {
                  shift-right: [w237] -> _
                  shift-left: w222 -> [w240]
                  shift-right: [w238] -> w233
                  shift-left: w221 -> [w239]
                  tunnel: w232 -> [w236]
                  stop <- w243 stop-if-true
                  w242 = u16 2 items=["microsteps", "microns", "millimeters", "inches"] ("Units (0: microsteps)")
                  n165 = Unbundle(w236) -> ("Microstep Size"=w235:dbl, "Device"=w234:string)
                  n166 = Wait (ms)(milliseconds to wait=u32 100) -> ()  [unwired: 1 out]
                  n167 = call "Read Current Position.vi"("Units (0: microsteps)"=w242, "error in (no error)"=w239, "Device and Axis"=w234, "Microstep Size (0)"=w235, "VISA resource name"=w240) -> ("error out"=w238:errorcluster, "Position"=w241:dbl, "VISA resource name out"=w237:refnum<visa-resource-name>)  [unwired: 4 in]
                  n168 = Not(x="Up") -> (.not. x?=w243:bool)
                  n169 = local write "Y [mm]"(w241) -> ()
                }
                n170 = local write "ZaberError"(w233) -> ()
              }
            }
          }
          event "GoToY": Value Change {
            w247 = u16 2 items=["device units", "microns/s^2", "mm/s^2", "inches/s^2", "degrees/s^2"] ("Units (0: data)")
            w256 = u16 2 items=["device speed units", "microns per second", "millimeters per second", "inches per second", "degrees per second"] ("Units (0: device speed units)")
            w262 = u16 2 items=["microsteps", "microns", "millimeters", "inches", "degrees"] ("Units (0: microsteps)")
            w265 = u16 1 items=["relative", "absolute"] ("Movement Type (0: relative)")
            n171 = event-data() -> ()  [unwired: 1 in, 6 out]
            n172 = local read "Assignment"() -> (w261:cluster{"Microstep Size":dbl, "Device":string}[])
            n173 = Index Array(array=w261, index=1) -> (element=w258:cluster{"Microstep Size":dbl, "Device":string})
            n174 = local read "Port"() -> (w254:refnum<visa-resource-name>)
            n175 = local read "ZaberError"() -> (w257:errorcluster)
            n176 = local read "XY Speed\n[mm/s]"() -> (w255:dbl)
            n177 = Unbundle(w258) -> ("Microstep Size"=w253:dbl, "Device"=w252:string)
            n178 = local read "Acceleration [mm/s^2]"() -> (w246:dbl)
            n179 = call "Set Speed.vi"("Units (0: data)"=w256, "New Speed"=w255, "error in (no error)"=w257, "Device and Axis"=w252, "Microstep Size (0)"=w253, "VISA resource name"=w254) -> ("error out"=w251:errorcluster, "VISA resource name out"=w249:refnum<visa-resource-name>)  [unwired: 4 in]
            n180 = call "Set Acceleration.vi"("Units (0: data)"=w247, "New Acceleration"=w246, "error in (no error)"=w251, "Device and Axis"=w252, "Microstep Size (0)"=w253, "VISA resource name"=w249) -> ("error out"=w250:errorcluster, "VISA resource name out"=w248:refnum<visa-resource-name>)  [unwired: 4 in]
            n181 = Unbundle(w258) -> ("Microstep Size"=w260:dbl, "Device"=w259:string)
            n182 = call "Move.vi"("Units (0: microsteps)"=w262, "Movement Type (0: relative)"=w265, "Move Distance (0)"="GoTo Y [mm]", "error in (no error)"=w250, "Device and Axis"=w259, "Microstep Size (0)"=w260, "VISA resource name"=w248) -> ("error out"=w263:errorcluster)  [unwired: 3 in, 1 out]
            n183 = local write "ZaberError"(w263) -> ()
          }
          event "GoToX": Value Change {
            w270 = u16 2 items=["device units", "microns/s^2", "mm/s^2", "inches/s^2", "degrees/s^2"] ("Units (0: data)")
            w281 = u16 2 items=["device speed units", "microns per second", "millimeters per second", "inches per second", "degrees per second"] ("Units (0: device speed units)")
            w285 = u16 2 items=["microsteps", "microns", "millimeters", "inches", "degrees"] ("Units (0: microsteps)")
            w287 = u16 1 items=["relative", "absolute"] ("Movement Type (0: relative)")
            # "move to point command"
            n184 = event-data() -> ()  [unwired: 1 in, 6 out]
            n185 = local read "Assignment"() -> (w280:cluster{"Microstep Size":dbl, "Device":string}[])
            n186 = local read "XY Speed\n[mm/s]"() -> (w283:dbl)
            n187 = local read "Port"() -> (w282:refnum<visa-resource-name>)
            n188 = Index Array(array=w280, index=0) -> (element=w277:cluster{"Microstep Size":dbl, "Device":string})
            n189 = local read "ZaberError"() -> (w284:errorcluster)
            n190 = Unbundle(w277) -> ("Microstep Size"=w272:dbl, "Device"=w271:string)
            n191 = local read "Acceleration [mm/s^2]"() -> (w269:dbl)
            n192 = call "Set Speed.vi"("Units (0: data)"=w281, "New Speed"=w283, "error in (no error)"=w284, "Device and Axis"=w271, "Microstep Size (0)"=w272, "VISA resource name"=w282) -> ("error out"=w274:errorcluster, "VISA resource name out"=w276:refnum<visa-resource-name>)  [unwired: 4 in]
            n193 = call "Set Acceleration.vi"("Units (0: data)"=w270, "New Acceleration"=w269, "error in (no error)"=w274, "Device and Axis"=w271, "Microstep Size (0)"=w272, "VISA resource name"=w276) -> ("error out"=w273:errorcluster, "VISA resource name out"=w275:refnum<visa-resource-name>)  [unwired: 4 in]
            n194 = Unbundle(w277) -> ("Microstep Size"=w279:dbl, "Device"=w278:string)
            n195 = call "Move.vi"("Units (0: microsteps)"=w285, "Movement Type (0: relative)"=w287, "Move Distance (0)"="GoTo X [mm]", "error in (no error)"=w273, "Device and Axis"=w278, "Microstep Size (0)"=w279, "VISA resource name"=w275) -> ("error out"=w286:errorcluster)  [unwired: 3 in, 1 out]
            n196 = local write "ZaberError"(w286) -> ()
          }
          event "GoToZ": Value Change {
            w299 = u16 2 items=["device units", "microns/s^2", "mm/s^2", "inches/s^2", "degrees/s^2"] ("Units (0: data)")
            w301 = u16 2 items=["device speed units", "microns per second", "millimeters per second", "inches per second", "degrees per second"] ("Units (0: device speed units)")
            w308 = u16 2 items=["microsteps", "microns", "millimeters", "inches", "degrees"] ("Units (0: microsteps)")
            w311 = u16 1 items=["relative", "absolute"] ("Movement Type (0: relative)")
            # "move to point command"
            n197 = event-data() -> ()  [unwired: 1 in, 6 out]
            n198 = local read "Assignment"() -> (w307:cluster{"Microstep Size":dbl, "Device":string}[])
            n199 = local read "ZaberError"() -> (w300:errorcluster)
            n200 = Index Array(array=w307, index=2) -> (element=w306:cluster{"Microstep Size":dbl, "Device":string})
            n201 = local read "Speed Z [mm/s]"() -> (w302:dbl)
            n202 = local read "Port"() -> (w303:refnum<visa-resource-name>)
            n203 = Unbundle(w306) -> ("Microstep Size"=w293:dbl, "Device"=w294:string)
            n204 = call "Set Speed.vi"("Units (0: data)"=w301, "New Speed"=w302, "error in (no error)"=w300, "Device and Axis"=w294, "Microstep Size (0)"=w293, "VISA resource name"=w303) -> ("error out"=w296:errorcluster, "VISA resource name out"=w298:refnum<visa-resource-name>)  [unwired: 4 in]
            n205 = local read "Acceleration [mm/s^2]"() -> (w292:dbl)
            n206 = call "Set Acceleration.vi"("Units (0: data)"=w299, "New Acceleration"=w292, "error in (no error)"=w296, "Device and Axis"=w294, "Microstep Size (0)"=w293, "VISA resource name"=w298) -> ("error out"=w295:errorcluster, "VISA resource name out"=w297:refnum<visa-resource-name>)  [unwired: 4 in]
            n207 = Unbundle(w306) -> ("Microstep Size"=w305:dbl, "Device"=w304:string)
            n208 = call "Move.vi"("Units (0: microsteps)"=w308, "Movement Type (0: relative)"=w311, "Move Distance (0)"="GoTo Z [mm]", "error in (no error)"=w295, "Device and Axis"=w304, "Microstep Size (0)"=w305, "VISA resource name"=w297) -> ("error out"=w310:errorcluster)  [unwired: 3 in, 1 out]
            n209 = local write "ZaberError"(w310) -> ()
          }
          event "StopMotion": Value Change {
            # "stop command"
            n210 = event-data() -> ()  [unwired: 1 in, 6 out]
            n211 = local read "Assignment"() -> (w318:cluster{"Microstep Size":dbl, "Device":string}[])
            n212 = local read "ZaberError"() -> (w316:errorcluster)
            n213 = local read "Port"() -> (w317:refnum<visa-resource-name>)
            n214 = for {
              tunnel: w318 -> [w322] mode=indexing
              shift-right: [w323] -> _
              shift-left: w317 -> [w326]
              shift-right: [w324] -> w315
              shift-left: w316 -> [w325]
              n215 = Unbundle(w322) -> ("Device"=w321:string)  [unwired: 1 out]
              n216 = call "Stop.vi"("error in (no error)"=w325, "Device and Axis"=w321, "VISA resource name"=w326) -> ("error out"=w324:errorcluster, "VISA resource name out"=w323:refnum<visa-resource-name>)  [unwired: 7 in]
            }
            n217 = local write "ZaberError"(w315) -> ()
          }
          event "Down": Value Change {
            n218 = event-data() -> ("NewVal"=w330:bool)  [unwired: 1 in, 5 out]
            n219 = local read "Assignment"() -> (w327:cluster{"Microstep Size":dbl, "Device":string}[])
            n220 = Index Array(array=w327, index=1) -> (element=w328:cluster{"Microstep Size":dbl, "Device":string})
            n221 = case shown="True" w330 {
              tunnel: w328 -> [_ w348]
              frame False {
                # "stop command"
                n222 = local read "Port"() -> (w335:refnum<visa-resource-name>)
                n223 = local read "ZaberError"() -> (w334:errorcluster)
                n224 = call "Stop.vi"("error in (no error)"=w334, "VISA resource name"=w335) -> ("error out"=w333:errorcluster)  [unwired: 8 in, 1 out]
                n225 = local write "ZaberError"(w333) -> ()
              }
              frame True {
                w347 = u16 2 items=["device units", "microns/s^2", "mm/s^2", "inches/s^2", "degrees/s^2"] ("Units (0: data)")
                w338 = u16 2 items=["device speed units", "microns per second", "millimeters per second", "inches per second", "degrees per second"] ("Units (0: device speed units)")
                # "move at specified velocity command"
                n226 = local read "Acceleration [mm/s^2]"() -> (w346:dbl)
                n227 = local read "ZaberError"() -> (w344:errorcluster)
                n228 = local read "Port"() -> (w345:refnum<visa-resource-name>)
                n229 = local read "XY Speed\n[mm/s]"() -> (w339:dbl)
                n230 = Unbundle(w348) -> ("Microstep Size"=w336:dbl, "Device"=w337:string)
                n231 = call "Set Acceleration.vi"("Units (0: data)"=w347, "New Acceleration"=w346, "error in (no error)"=w344, "Device and Axis"=w337, "Microstep Size (0)"=w336, "VISA resource name"=w345) -> ("error out"=w342:errorcluster, "VISA resource name out"=w343:refnum<visa-resource-name>)  [unwired: 4 in]
                n232 = call "Move at Velocity.vi"("Units (0: device speed units)"=w338, "Velocity"=w339, "error in (no error)"=w342, "Device and Axis"=w337, "Microstep Size (0)"=w336, "VISA resource name"=w343) -> ("error out"=w340:errorcluster, "VISA resource name out"=w341:refnum<visa-resource-name>)  [unwired: 4 in]
                n233 = while {
                  shift-right: [w354] -> _
                  shift-left: w341 -> [w357]
                  shift-right: [w355] -> w349
                  shift-left: w340 -> [w356]
                  tunnel: w348 -> [w350]
                  stop <- w360 stop-if-true
                  w359 = u16 2 items=["microsteps", "microns", "millimeters", "inches"] ("Units (0: microsteps)")
                  n234 = Wait (ms)(milliseconds to wait=u32 100) -> ()  [unwired: 1 out]
                  n235 = Unbundle(w350) -> ("Microstep Size"=w352:dbl, "Device"=w351:string)
                  n236 = call "Read Current Position.vi"("Units (0: microsteps)"=w359, "error in (no error)"=w356, "Device and Axis"=w351, "Microstep Size (0)"=w352, "VISA resource name"=w357) -> ("error out"=w355:errorcluster, "Position"=w358:dbl, "VISA resource name out"=w354:refnum<visa-resource-name>)  [unwired: 4 in]
                  n237 = Not(x="Down") -> (.not. x?=w360:bool)
                  n238 = local write "Y [mm]"(w358) -> ()
                }
                n239 = local write "ZaberError"(w349) -> ()
              }
            }
          }
          event "Closer": Value Change {
            n240 = event-data() -> ("NewVal"=w363:bool)  [unwired: 1 in, 5 out]
            n241 = local read "Assignment"() -> (w362:cluster{"Microstep Size":dbl, "Device":string}[])
            n242 = Index Array(array=w362, index=2) -> (element=w364:cluster{"Microstep Size":dbl, "Device":string})
            n243 = case shown="True" w363 {
              tunnel: w364 -> [_ w383]
              frame False {
                # "stop command"
                n244 = local read "Port"() -> (w370:refnum<visa-resource-name>)
                n245 = local read "ZaberError"() -> (w369:errorcluster)
                n246 = call "Stop.vi"("error in (no error)"=w369, "VISA resource name"=w370) -> ("error out"=w368:errorcluster)  [unwired: 8 in, 1 out]
                n247 = local write "ZaberError"(w368) -> ()
              }
              frame True {
                w381 = u16 2 items=["device units", "microns/s^2", "mm/s^2", "inches/s^2", "degrees/s^2"] ("Units (0: data)")
                w375 = u16 2 items=["device speed units", "microns per second", "millimeters per second", "inches per second", "degrees per second"] ("Units (0: device speed units)")
                # "move at specified velocity command"
                n248 = local read "Acceleration [mm/s^2]"() -> (w382:dbl)
                n249 = local read "ZaberError"() -> (w379:errorcluster)
                n250 = local read "Speed Z [mm/s]"() -> (w374:dbl)
                n251 = local read "Port"() -> (w380:refnum<visa-resource-name>)
                n252 = Unbundle(w383) -> ("Microstep Size"=w377:dbl, "Device"=w376:string)
                n253 = call "Set Acceleration.vi"("Units (0: data)"=w381, "New Acceleration"=w382, "error in (no error)"=w379, "Device and Axis"=w376, "Microstep Size (0)"=w377, "VISA resource name"=w380) -> ("error out"=w378:errorcluster, "VISA resource name out"=w372:refnum<visa-resource-name>)  [unwired: 4 in]
                n254 = call "Move at Velocity.vi"("Units (0: device speed units)"=w375, "Velocity"=w374, "error in (no error)"=w378, "Device and Axis"=w376, "Microstep Size (0)"=w377, "VISA resource name"=w372) -> ("error out"=w373:errorcluster, "VISA resource name out"=w371:refnum<visa-resource-name>)  [unwired: 4 in]
                n255 = while {
                  shift-right: [w390] -> _
                  shift-left: w371 -> [w393]
                  shift-right: [w391] -> w384
                  shift-left: w373 -> [w392]
                  tunnel: w383 -> [w385]
                  stop <- w395 stop-if-true
                  w394 = u16 2 items=["microsteps", "microns", "millimeters", "inches"] ("Units (0: microsteps)")
                  n256 = Wait (ms)(milliseconds to wait=u32 100) -> ()  [unwired: 1 out]
                  n257 = Unbundle(w385) -> ("Microstep Size"=w387:dbl, "Device"=w386:string)
                  n258 = call "Read Current Position.vi"("Units (0: microsteps)"=w394, "error in (no error)"=w392, "Device and Axis"=w386, "Microstep Size (0)"=w387, "VISA resource name"=w393) -> ("error out"=w391:errorcluster, "Position"=w389:dbl, "VISA resource name out"=w390:refnum<visa-resource-name>)  [unwired: 4 in]
                  n259 = Not(x="Closer") -> (.not. x?=w395:bool)
                  n260 = local write "Z [mm]"(w389) -> ()
                }
                n261 = local write "ZaberError"(w384) -> ()
              }
            }
          }
          event "Left": Value Change {
            n262 = event-data() -> ("NewVal"=w398:bool)  [unwired: 1 in, 5 out]
            n263 = local read "Assignment"() -> (w397:cluster{"Microstep Size":dbl, "Device":string}[])
            n264 = Index Array(array=w397, index=0) -> (element=w399:cluster{"Microstep Size":dbl, "Device":string})
            n265 = case shown="True" w398 {
              tunnel: w399 -> [_ w418]
              frame False {
                # "stop command"
                n266 = local read "Port"() -> (w405:refnum<visa-resource-name>)
                n267 = local read "ZaberError"() -> (w404:errorcluster)
                n268 = call "Stop.vi"("error in (no error)"=w404, "VISA resource name"=w405) -> ("error out"=w403:errorcluster)  [unwired: 8 in, 1 out]
                n269 = local write "ZaberError"(w403) -> ()
              }
              frame True {
                w417 = u16 2 items=["device units", "microns/s^2", "mm/s^2", "inches/s^2", "degrees/s^2"] ("Units (0: data)")
                w407 = u16 2 items=["device speed units", "microns per second", "millimeters per second", "inches per second", "degrees per second"] ("Units (0: device speed units)")
                # "move at specified velocity command"
                n270 = local read "ZaberError"() -> (w414:errorcluster)
                n271 = local read "XY Speed\n[mm/s]"() -> (w419:dbl)
                n272 = local read "Port"() -> (w415:refnum<visa-resource-name>)
                n273 = Negate(x=w419) -> (-x=w406:dbl)
                n274 = local read "Acceleration [mm/s^2]"() -> (w416:dbl)
                n275 = Unbundle(w418) -> ("Microstep Size"=w409:dbl, "Device"=w408:string)
                n276 = call "Set Acceleration.vi"("Units (0: data)"=w417, "New Acceleration"=w416, "error in (no error)"=w414, "Device and Axis"=w408, "Microstep Size (0)"=w409, "VISA resource name"=w415) -> ("error out"=w412:errorcluster, "VISA resource name out"=w413:refnum<visa-resource-name>)  [unwired: 4 in]
                n277 = call "Move at Velocity.vi"("Units (0: device speed units)"=w407, "Velocity"=w406, "error in (no error)"=w412, "Device and Axis"=w408, "Microstep Size (0)"=w409, "VISA resource name"=w413) -> ("error out"=w410:errorcluster, "VISA resource name out"=w411:refnum<visa-resource-name>)  [unwired: 4 in]
                n278 = while {
                  shift-right: [w426] -> _
                  shift-left: w411 -> [w429]
                  shift-right: [w427] -> w420
                  shift-left: w410 -> [w428]
                  tunnel: w418 -> [w423]
                  stop <- w431 stop-if-true
                  w430 = u16 2 items=["microsteps", "microns", "millimeters", "inches"] ("Units (0: microsteps)")
                  n279 = Unbundle(w423) -> ("Microstep Size"=w422:dbl, "Device"=w421:string)
                  n280 = Wait (ms)(milliseconds to wait=u32 100) -> ()  [unwired: 1 out]
                  n281 = call "Read Current Position.vi"("Units (0: microsteps)"=w430, "error in (no error)"=w428, "Device and Axis"=w421, "Microstep Size (0)"=w422, "VISA resource name"=w429) -> ("error out"=w427:errorcluster, "Position"=w425:dbl, "VISA resource name out"=w426:refnum<visa-resource-name>)  [unwired: 4 in]
                  n282 = Not(x="Left") -> (.not. x?=w431:bool)
                  n283 = local write "X [mm]"(w425) -> ()
                }
                n284 = local write "ZaberError"(w420) -> ()
              }
            }
          }
          event "Right": Value Change {
            n285 = event-data() -> ("NewVal"=w434:bool)  [unwired: 1 in, 5 out]
            n286 = local read "Assignment"() -> (w433:cluster{"Microstep Size":dbl, "Device":string}[])
            n287 = Index Array(array=w433, index=0) -> (element=w435:cluster{"Microstep Size":dbl, "Device":string})
            n288 = case shown="True" w434 {
              tunnel: w435 -> [_ w454]
              frame False {
                # "stop command"
                n289 = local read "Port"() -> (w441:refnum<visa-resource-name>)
                n290 = local read "ZaberError"() -> (w440:errorcluster)
                n291 = call "Stop.vi"("error in (no error)"=w440, "VISA resource name"=w441) -> ("error out"=w439:errorcluster)  [unwired: 8 in, 1 out]
                n292 = local write "ZaberError"(w439) -> ()
              }
              frame True {
                w453 = u16 2 items=["device units", "microns/s^2", "mm/s^2", "inches/s^2", "degrees/s^2"] ("Units (0: data)")
                w443 = u16 2 items=["device speed units", "microns per second", "millimeters per second", "inches per second", "degrees per second"] ("Units (0: device speed units)")
                # "move at specified velocity command"
                n293 = local read "Acceleration [mm/s^2]"() -> (w452:dbl)
                n294 = local read "ZaberError"() -> (w451:errorcluster)
                n295 = local read "XY Speed\n[mm/s]"() -> (w442:dbl)
                n296 = local read "Port"() -> (w450:refnum<visa-resource-name>)
                n297 = Unbundle(w454) -> ("Microstep Size"=w445:dbl, "Device"=w444:string)
                n298 = call "Set Acceleration.vi"("Units (0: data)"=w453, "New Acceleration"=w452, "error in (no error)"=w451, "Device and Axis"=w444, "Microstep Size (0)"=w445, "VISA resource name"=w450) -> ("error out"=w449:errorcluster, "VISA resource name out"=w448:refnum<visa-resource-name>)  [unwired: 4 in]
                n299 = call "Move at Velocity.vi"("Units (0: device speed units)"=w443, "Velocity"=w442, "error in (no error)"=w449, "Device and Axis"=w444, "Microstep Size (0)"=w445, "VISA resource name"=w448) -> ("error out"=w446:errorcluster, "VISA resource name out"=w447:refnum<visa-resource-name>)  [unwired: 4 in]
                n300 = while {
                  shift-right: [w461] -> _
                  shift-left: w447 -> [w464]
                  shift-right: [w462] -> w455
                  shift-left: w446 -> [w463]
                  tunnel: w454 -> [w456]
                  stop <- w466 stop-if-true
                  w465 = u16 2 items=["microsteps", "microns", "millimeters", "inches"] ("Units (0: microsteps)")
                  n301 = Wait (ms)(milliseconds to wait=u32 100) -> ()  [unwired: 1 out]
                  n302 = Unbundle(w456) -> ("Microstep Size"=w458:dbl, "Device"=w457:string)
                  n303 = call "Read Current Position.vi"("Units (0: microsteps)"=w465, "error in (no error)"=w463, "Device and Axis"=w457, "Microstep Size (0)"=w458, "VISA resource name"=w464) -> ("error out"=w462:errorcluster, "Position"=w460:dbl, "VISA resource name out"=w461:refnum<visa-resource-name>)  [unwired: 4 in]
                  n304 = Not(x="Right") -> (.not. x?=w466:bool)
                  n305 = local write "X [mm]"(w460) -> ()
                }
                n306 = local write "ZaberError"(w455) -> ()
              }
            }
          }
          event "Away": Value Change {
            n307 = event-data() -> ("NewVal"=w469:bool)  [unwired: 1 in, 5 out]
            n308 = local read "Assignment"() -> (w468:cluster{"Microstep Size":dbl, "Device":string}[])
            n309 = Index Array(array=w468, index=2) -> (element=w470:cluster{"Microstep Size":dbl, "Device":string})
            n310 = case shown="True" w469 {
              tunnel: w470 -> [_ w489]
              frame False {
                # "stop command"
                n311 = local read "Port"() -> (w476:refnum<visa-resource-name>)
                n312 = local read "ZaberError"() -> (w475:errorcluster)
                n313 = call "Stop.vi"("error in (no error)"=w475, "VISA resource name"=w476) -> ("error out"=w474:errorcluster)  [unwired: 8 in, 1 out]
                n314 = local write "ZaberError"(w474) -> ()
              }
              frame True {
                w488 = u16 2 items=["device units", "microns/s^2", "mm/s^2", "inches/s^2", "degrees/s^2"] ("Units (0: data)")
                w482 = u16 2 items=["device speed units", "microns per second", "millimeters per second", "inches per second", "degrees per second"] ("Units (0: device speed units)")
                # "move at specified velocity command"
                n315 = local read "Acceleration [mm/s^2]"() -> (w487:dbl)
                n316 = local read "Speed Z [mm/s]"() -> (w490:dbl)
                n317 = local read "Port"() -> (w485:refnum<visa-resource-name>)
                n318 = local read "ZaberError"() -> (w486:errorcluster)
                n319 = Negate(x=w490) -> (-x=w481:dbl)
                n320 = Unbundle(w489) -> ("Microstep Size"=w484:dbl, "Device"=w483:string)
                n321 = call "Set Acceleration.vi"("Units (0: data)"=w488, "New Acceleration"=w487, "error in (no error)"=w486, "Device and Axis"=w483, "Microstep Size (0)"=w484, "VISA resource name"=w485) -> ("error out"=w479:errorcluster, "VISA resource name out"=w480:refnum<visa-resource-name>)  [unwired: 4 in]
                n322 = call "Move at Velocity.vi"("Units (0: device speed units)"=w482, "Velocity"=w481, "error in (no error)"=w479, "Device and Axis"=w483, "Microstep Size (0)"=w484, "VISA resource name"=w480) -> ("error out"=w478:errorcluster, "VISA resource name out"=w477:refnum<visa-resource-name>)  [unwired: 4 in]
                n323 = while {
                  shift-right: [w497] -> _
                  shift-left: w477 -> [w500]
                  shift-right: [w498] -> w491
                  shift-left: w478 -> [w499]
                  tunnel: w489 -> [w494]
                  stop <- w502 stop-if-true
                  w501 = u16 2 items=["microsteps", "microns", "millimeters", "inches"] ("Units (0: microsteps)")
                  n324 = Unbundle(w494) -> ("Microstep Size"=w493:dbl, "Device"=w492:string)
                  n325 = Wait (ms)(milliseconds to wait=u32 100) -> ()  [unwired: 1 out]
                  n326 = call "Read Current Position.vi"("Units (0: microsteps)"=w501, "error in (no error)"=w499, "Device and Axis"=w492, "Microstep Size (0)"=w493, "VISA resource name"=w500) -> ("error out"=w498:errorcluster, "Position"=w496:dbl, "VISA resource name out"=w497:refnum<visa-resource-name>)  [unwired: 4 in]
                  n327 = Not(x="Away") -> (.not. x?=w502:bool)
                  n328 = local write "Z [mm]"(w496) -> ()
                }
                n329 = local write "ZaberError"(w491) -> ()
              }
            }
          }
          event "Reduced Speed": Value Change {
            n330 = event-data() -> ("NewVal"=w518:bool)  [unwired: 1 in, 5 out]
            n331 = case shown="False" w518 {
              tunnel: [1.0 ("Minimum") 0.1 ("Minimum")] -> w515
              tunnel: [75.0 ("Minimum") 7.5 ("Minimum")] -> w514
              tunnel: [1.0 ("Minimum") 0.1 ("Minimum")] -> w513
              tunnel: [0.5 ("Minimum") 0.05 ("Minimum")] -> w506
              tunnel: [10.0 ("Minimum") 1.0 ("Minimum")] -> w505
              tunnel: [0.5 ("Minimum") 0.05 ("Minimum")] -> w504
              frame False {
                # "full speed"
              }
              frame True {
                # "reduced speed"
              }
            }
            n332 = property on="Speed Z [mm/s]" class="Slide (strict)"() -> ("Data Range"=w508:T11, "Scale.Range"=w507:T12)  [unwired: 2 in, 2 out]
            n333 = property on="XY Speed\n[mm/s]" class="Slide (strict)"() -> ("Data Range"=w520:T11, "Scale.Range"=w512:T12)  [unwired: 2 in, 2 out]
            n334 = Bundle By Name(cluster=w520, "Minimum"=w515, "Maximum"=w514, "Increment"=w513) -> (w519:T11)
            n335 = Bundle By Name(cluster=w512, "Minimum"=w515, "Maximum"=w514, "Increment"=w513) -> (w511:T12)
            n336 = Bundle By Name(cluster=w508, "Minimum"=w506, "Maximum"=w505, "Increment"=w504) -> (w510:T11)
            n337 = Bundle By Name(cluster=w507, "Minimum"=w506, "Maximum"=w505, "Increment"=w504) -> (w509:T12)
            n338 = property on="XY Speed\n[mm/s]" class="Slide (strict)"("Data Range"=w519, "Scale.Range"=w511) -> ()  [unwired: 2 in, 2 out]
            n339 = property on="Speed Z [mm/s]" class="Slide (strict)"("Data Range"=w510, "Scale.Range"=w509) -> ()  [unwired: 2 in, 2 out]
          }
          event Panel Close? {
            n340 = event-data() -> ()  [unwired: 1 in, 4 out]
            n341 = local read "DANTE configured"() -> (w534:bool)
            n342 = case shown="True" w534 {
              tunnel: [fast_scanner."Close" ("Enum") fast_scanner."IDLE" ("Enum")] -> w533
              frame False {
              }
              frame True {
                n343 = One Button Dialog(message="Close DANTE first") -> ()  [unwired: 1 in, 1 out]
              }
            }
            n344 = event-data("Discard?"=TRUE) -> ()  [unwired: 1 in, 1 out]
          }
          event "MEASUREMENT_Start": Value Change {
            n345 = event-data() -> ()  [unwired: 1 in, 5 out]
          }
          event "SpectraPlot": Mouse Up {
            (unwired) FALSE
            n346 = event-data() -> ()  [unwired: 1 in, 8 out]
            n347 = control-ref of="SpectraPlot"() -> (w547:refnum<vi>)
            n348 = property class="WFGraph (strict)"(reference=w547, "Active Cursor"=u32 1, "Active Cursor"=u32 2) -> ("Cursor.Cursor X"=w544:dbl, "Cursor.Cursor X"=w545:dbl)  [unwired: 1 in, 2 out]
            n349 = Less?(x=w544, y=w545) -> (x < y?=w546:bool)
            n350 = case shown="False" w546 {
              tunnel: w544 -> [w552 w555]
              tunnel: w545 -> [w553 w554]
              tunnel: [w553 w555] -> w548
              tunnel: [w552 w554] -> w549
              frame False {
              }
              frame True {
              }
            }
            "ROI Begin" <- w548
            "ROI End" <- w549
          }
          event "APPEARANCE_CursorVis": Value Change {
            n351 = event-data() -> ("NewVal"=w557:bool)  [unwired: 1 in]
            n352 = property on="SpectraPlot" class="WFGraph (strict)"("Cursor Palette Vis"=w557, "Active Cursor"=u32 0, "Cursor.Visible"=w557) -> ()  [unwired: 2 in, 2 out]
          }
          event "APPEARANCE_Log/Lin": Value Change {
            n353 = event-data() -> ("NewVal"=w562:bool)  [unwired: 1 in]
            n354 = Boolean To (0,1)(Boolean=w562) -> (0, 1=w561:i16)
            n355 = property on="SpectraPlot" class="WFGraph (strict)"("YScale.Mapping Mode"=w561) -> ()  [unwired: 2 in, 2 out]
          }
        }
      }
      frame "Acquire" {
        # "if not mapping plot last spectra on spectra plot"
        n356 = local read "identifier out"() -> (w569:string)
        n357 = Multiply(x="Preset Time [s]", y=10.0) -> (x*y=w564:dbl)
        n358 = control-ref of="SpectraPlot"() -> (w567:refnum<vi>)
        n359 = call "DANTE acquire single.vi"("Ctl Refnum"=w567, "Acquisition time [s]"=w564, "identifier out"=w569) -> ("stats out"=→"stats out":T5)  [unwired: 7 in, 1 out]
      }
      frame "PrepareMap" {
        n360 = local read "X start [mm]"() -> (w586:dbl)
        n361 = local read "Y start [mm]"() -> (w591:dbl)
        n362 = local read "step Y [mm]"() -> (w588:dbl)
        n363 = local read "X [mm]"() -> (w585:dbl)
        n364 = local read "Y [mm]"() -> (w590:dbl)
        n365 = local read "X end [mm]"() -> (w581:dbl)
        n366 = local read "X [mm]"() -> (w580:dbl)
        n367 = local read "Y steps"() -> (w578:i32)
        "total line #" <- w578
        n368 = Add(x=w586, y=w585) -> (x+y=→"X start position":dbl)
        n369 = Add(x=w581, y=w580) -> (x+y=→"X end position":dbl)
        n370 = Add(x=w590, y=w591) -> (x+y=w589:dbl)
        n371 = for {
          N: w578 -> [_]
          tunnel: w589 -> [w599]
          tunnel: w588 -> [w600]
          tunnel: [w597] -> w587 mode=indexing
          i -> [w601]
          n372 = Multiply(x=w600, y=w601) -> (x*y=w598:dbl)
          n373 = Add(x=w599, y=w598) -> (x+y=w597:dbl)
        }
        "Y positions array" <- w587
        n374 = local read "X steps"() -> (w575:i32)
        n375 = local read "Y steps"() -> (w573:i32)
        n376 = Increment(x=w573) -> (x+1=w572:i32)
        n377 = Initialize Array(u32 0 ("element"), w575, w572) -> (→"ROI map":u32[][])
        n378 = for {
          N: w578 -> [_]
          tunnel: [w594] -> w577 mode=indexing
          n379 = Initialize Array(0.0 ("element"), 4 ("dimension size")) -> (w594:dbl[])
        }
        "scan timing [ms]" <- w577
        "scan mode" <- TRUE ("scan mode")
        "Line #" <- 1 ("Line #")
      }
      frame "MoveToStartPoint" {
        n380 = stacked-sequence {
          frame #0 {
            w610 = u16 2 items=["device units", "microns/s^2", "mm/s^2", "inches/s^2", "degrees/s^2"] ("Units (0: data)")
            w618 = u16 2 items=["device speed units", "microns per second", "millimeters per second", "inches per second", "degrees per second"] ("Units (0: device speed units)")
            w624 = u16 2 items=["microsteps", "microns", "millimeters", "inches", "degrees"] ("Units (0: microsteps)")
            w626 = u16 1 items=["relative", "absolute"] ("Movement Type (0: relative)")
            n381 = local read "Line #"() -> (w605:i32)
            n382 = local read "Y positions array"() -> (w609:dbl[])
            n383 = local read "Assignment"() -> (w623:cluster{"Microstep Size":dbl, "Device":string}[])
            n384 = Decrement(x=w605) -> (x-1=w604:i32)
            n385 = Index Array(array=w609, index=w604) -> (element=w608:dbl)
            n386 = Index Array(array=w623, index=1) -> (element=w620:cluster{"Microstep Size":dbl, "Device":string})
            n387 = local read "Port"() -> (w617:refnum<visa-resource-name>)
            n388 = local read "ZaberError"() -> (w619:errorcluster)
            n389 = local read "X velocity [mm/s]"() -> (w606:dbl)
            n390 = Unbundle(w620) -> ("Microstep Size"=w616:dbl, "Device"=w615:string)
            n391 = call "Set Speed.vi"("Units (0: data)"=w618, "New Speed"=w606, "error in (no error)"=w619, "Device and Axis"=w615, "Microstep Size (0)"=w616, "VISA resource name"=w617) -> ("error out"=w614:errorcluster, "VISA resource name out"=w612:refnum<visa-resource-name>)  [unwired: 4 in]
            n392 = local read "X accel"() -> (w607:dbl)
            n393 = call "Set Acceleration.vi"("Units (0: data)"=w610, "New Acceleration"=w607, "error in (no error)"=w614, "Device and Axis"=w615, "Microstep Size (0)"=w616, "VISA resource name"=w612) -> ("error out"=w613:errorcluster, "VISA resource name out"=w611:refnum<visa-resource-name>)  [unwired: 4 in]
            n394 = Unbundle(w620) -> ("Microstep Size"=w622:dbl, "Device"=w621:string)
            n395 = call "Move.vi"("Units (0: microsteps)"=w624, "Movement Type (0: relative)"=w626, "Move Distance (0)"=w608, "error in (no error)"=w613, "Device and Axis"=w621, "Microstep Size (0)"=w622, "VISA resource name"=w611) -> ("error out"=w625:errorcluster)  [unwired: 3 in, 1 out]
            n396 = local write "ZaberError"(w625) -> ()
          }
          frame #1 {
            w633 = u16 2 items=["device units", "microns/s^2", "mm/s^2", "inches/s^2", "degrees/s^2"] ("Units (0: data)")
            w644 = u16 2 items=["device speed units", "microns per second", "millimeters per second", "inches per second", "degrees per second"] ("Units (0: device speed units)")
            w647 = u16 2 items=["microsteps", "microns", "millimeters", "inches", "degrees"] ("Units (0: microsteps)")
            w649 = u16 1 items=["relative", "absolute"] ("Movement Type (0: relative)")
            # "move to point command"
            n397 = local read "Assignment"() -> (w643:cluster{"Microstep Size":dbl, "Device":string}[])
            n398 = local read "Port"() -> (w645:refnum<visa-resource-name>)
            n399 = Index Array(array=w643, index=0) -> (element=w640:cluster{"Microstep Size":dbl, "Device":string})
            n400 = local read "ZaberError"() -> (w646:errorcluster)
            n401 = local read "X velocity [mm/s]"() -> (w628:dbl)
            n402 = Unbundle(w640) -> ("Microstep Size"=w635:dbl, "Device"=w634:string)
            n403 = call "Set Speed.vi"("Units (0: data)"=w644, "New Speed"=w628, "error in (no error)"=w646, "Device and Axis"=w634, "Microstep Size (0)"=w635, "VISA resource name"=w645) -> ("error out"=w637:errorcluster, "VISA resource name out"=w639:refnum<visa-resource-name>)  [unwired: 4 in]
            n404 = local read "X start position"() -> (w632:dbl)
            n405 = local read "Acc dist [mm]"() -> (w631:dbl)
            n406 = local read "X accel"() -> (w629:dbl)
            n407 = call "Set Acceleration.vi"("Units (0: data)"=w633, "New Acceleration"=w629, "error in (no error)"=w637, "Device and Axis"=w634, "Microstep Size (0)"=w635, "VISA resource name"=w639) -> ("error out"=w636:errorcluster, "VISA resource name out"=w638:refnum<visa-resource-name>)  [unwired: 4 in]
            n408 = Subtract(x=w632, y=w631) -> (x-y=w630:dbl)
            n409 = Unbundle(w640) -> ("Microstep Size"=w642:dbl, "Device"=w641:string)
            n410 = call "Move.vi"("Units (0: microsteps)"=w647, "Movement Type (0: relative)"=w649, "Move Distance (0)"=w630, "error in (no error)"=w636, "Device and Axis"=w641, "Microstep Size (0)"=w642, "VISA resource name"=w638) -> ("error out"=w648:errorcluster)  [unwired: 3 in, 1 out]
            n411 = local write "ZaberError"(w648) -> ()
          }
          frame #2 {
            n412 = disable-structure shown="Enabled" {
              frame Disabled {
                # "wait till movement is completed"
                n413 = while {
                  stop <- w666 stop-if-true
                  w675 = u16 2 items=["microsteps", "microns", "millimeters", "inches"] ("Units (0: microsteps)")
                  # "Y"
                  # "X"
                  n414 = local read "Assignment"() -> (w676:cluster{"Microstep Size":dbl, "Device":string}[])
                  n415 = local read "ZaberError"() -> (w670:errorcluster)
                  n416 = local read "Port"() -> (w669:refnum<visa-resource-name>)
                  n417 = local read "X start position"() -> (w656:dbl)
                  n418 = local read "Acc dist [mm]"() -> (w655:dbl)
                  n419 = Index Array(array=w676, index=0) -> (element=w677:cluster{"Microstep Size":dbl, "Device":string})
                  n420 = Index Array(array=w676, index=1) -> (element=w678:cluster{"Microstep Size":dbl, "Device":string})
                  n421 = Subtract(x=w656, y=w655) -> (x-y=w654:dbl)
                  n422 = Unbundle(w677) -> ("Microstep Size"=w661:dbl, "Device"=w662:string)
                  n423 = call "Read Current Position.vi"("Units (0: microsteps)"=w675, "error in (no error)"=w670, "Device and Axis"=w662, "Microstep Size (0)"=w661, "VISA resource name"=w669) -> ("error out"=w671:errorcluster, "Position"=w660:dbl, "VISA resource name out"=w672:refnum<visa-resource-name>)  [unwired: 4 in]
                  n424 = local read "Y positions array"() -> (w652:dbl[])
                  n425 = call "ChkOnTarget.vi"("Prec"="Precision [mm]", "TargetPos"=w654, "CurrPos"=w660) -> ("In Range?"=w667:bool)
                  n426 = local read "Line #"() -> (w653:i32)
                  n427 = Unbundle(w678) -> ("Microstep Size"=w658:dbl, "Device"=w659:string)
                  n428 = Index Array(array=w652, index=w653) -> (element=w651:dbl)
                  n429 = call "Read Current Position.vi"("Units (0: microsteps)"=w675, "error in (no error)"=w671, "Device and Axis"=w659, "Microstep Size (0)"=w658, "VISA resource name"=w672) -> ("error out"=w664:errorcluster, "Position"=w657:dbl, "VISA resource name out"=w663:refnum<visa-resource-name>)  [unwired: 4 in]
                  n430 = call "ChkOnTarget.vi"("Prec"="Precision [mm]", "TargetPos"=w651, "CurrPos"=w657) -> ("In Range?"=w668:bool)
                  n431 = local write "Port"(w663) -> ()
                  n432 = local write "ZaberError"(w664) -> ()
                  n433 = Compound Arithmetic op=AND(w668, w667) -> (w666:bool)
                }
              }
              frame Enabled {
              }
            }
          }
          frame #3 {
            # "wait till movement is completed"
            n434 = local read "Assignment"() -> (w681:cluster{"Microstep Size":dbl, "Device":string}[])
            n435 = local read "ZaberError"() -> (w684:errorcluster)
            n436 = local read "Port"() -> (w685:refnum<visa-resource-name>)
            n437 = Index Array(array=w681, index=0) -> (element=w682:cluster{"Microstep Size":dbl, "Device":string})
            n438 = Index Array(array=w681, index=1) -> (element=w683:cluster{"Microstep Size":dbl, "Device":string})
            n439 = Unbundle(w682) -> ("Device"=w686:string)  [unwired: 1 out]
            n440 = call "Poll Until Idle.vi"("error in (no error)"=w684, "Device and Axis"=w686, "VISA resource name"=w685) -> ("error out"=w688:errorcluster, "VISA resource name out"=w691:refnum<visa-resource-name>)  [unwired: 7 in]
            n441 = Unbundle(w683) -> ("Device"=w687:string)  [unwired: 1 out]
            n442 = call "Poll Until Idle.vi"("error in (no error)"=w688, "Device and Axis"=w687, "VISA resource name"=w691) -> ("error out"=w689:errorcluster, "VISA resource name out"=w690:refnum<visa-resource-name>)  [unwired: 7 in]
            n443 = local write "Port"(w690) -> ()
            n444 = local write "ZaberError"(w689) -> ()
          }
        }
      }
      frame "AcquireLine" {
        # "stats"
        # "spectra"
        # "acceleration"
        # "waiting till movement completed"
        # "acquisition command"
        # "sending movement command"
        n445 = stacked-sequence {
          seq-local: [w694 _ _ _ _ _ _ _ _ _ _ _] -> [_ _ w719 _ _ _ _ _ _ _ _ _]
          seq-local: [_ _ w720 _ _ _ _ _ _ _ _ _] -> [_ _ _ _ w727 _ _ _ _ _ _ _]
          seq-local: [_ _ _ _ w728 _ _ _ _ _ _ _] -> [_ _ _ _ _ _ w740 _ _ _ _ _]
          seq-local: [_ _ w718 _ _ _ _ _ _ _ _ _] -> [_ _ _ _ _ _ _ _ _ _ _ w787]
          seq-local: [_ _ _ _ _ _ w739 _ _ _ _ _] -> [_ _ _ _ _ _ _ _ _ _ _ w785]
          seq-local: [_ _ _ _ _ _ w738 _ _ _ _ _] -> [_ _ _ _ _ _ _ _ w749 _ _ _]
          seq-local: [_ _ _ _ _ _ _ _ w748 _ _ _] -> [_ _ _ _ _ _ _ _ _ _ _ w784]
          seq-local: [_ _ _ _ w726 _ _ _ _ _ _ _] -> [_ _ _ _ _ _ _ _ _ _ _ w786]
          seq-local: [_ _ _ _ _ w734 _ _ _ _ _ _] -> [_ _ _ _ _ _ _ _ _ w758 w776 _]
          seq-local: [_ _ _ _ _ w733 _ _ _ _ _ _] -> [_ _ _ _ _ _ _ _ _ _ w774 _]
          seq-local: [_ _ _ _ _ w729 _ _ _ _ _ _] -> [_ _ _ _ _ _ _ _ _ _ w759 _]
          frame #0 {
            n446 = Tick Count (ms)() -> (millisecond timer value=w694:u32)
          }
          frame #1 {
            w717 = u16 2 items=["device units", "microns/s^2", "mm/s^2", "inches/s^2", "degrees/s^2"] ("Units (0: data)")
            w706 = u16 2 items=["device speed units", "microns per second", "millimeters per second", "inches per second", "degrees per second"] ("Units (0: device speed units)")
            w703 = u16 2 items=["microsteps", "microns", "millimeters", "inches", "degrees"] ("Units (0: microsteps)")
            w701 = u16 1 items=["relative", "absolute"] ("Movement Type (0: relative)")
            n447 = local read "Assignment"() -> (w707:cluster{"Microstep Size":dbl, "Device":string}[])
            n448 = local read "Port"() -> (w705:refnum<visa-resource-name>)
            n449 = Index Array(array=w707, index=0) -> (element=w710:cluster{"Microstep Size":dbl, "Device":string})
            n450 = local read "ZaberError"() -> (w704:errorcluster)
            n451 = local read "X scan velocity [mm/s]"() -> (w699:dbl)
            n452 = local read "X accel"() -> (w698:dbl)
            n453 = Unbundle(w710) -> ("Microstep Size"=w715:dbl, "Device"=w716:string)
            n454 = call "Set Speed.vi"("Units (0: data)"=w706, "New Speed"=w699, "error in (no error)"=w704, "Device and Axis"=w716, "Microstep Size (0)"=w715, "VISA resource name"=w705) -> ("error out"=w713:errorcluster, "VISA resource name out"=w711:refnum<visa-resource-name>)  [unwired: 4 in]
            n455 = local read "Acc dist [mm]"() -> (w695:dbl)
            n456 = local read "X end position"() -> (w696:dbl)
            n457 = call "Set Acceleration.vi"("Units (0: data)"=w717, "New Acceleration"=w698, "error in (no error)"=w713, "Device and Axis"=w716, "Microstep Size (0)"=w715, "VISA resource name"=w711) -> ("error out"=w714:errorcluster, "VISA resource name out"=w712:refnum<visa-resource-name>)  [unwired: 4 in]
            n458 = Add(x=w696, y=w695) -> (x+y=w697:dbl)
            n459 = Unbundle(w710) -> ("Microstep Size"=w708:dbl, "Device"=w709:string)
            n460 = call "Move.vi"("Units (0: microsteps)"=w703, "Movement Type (0: relative)"=w701, "Move Distance (0)"=w697, "error in (no error)"=w714, "Device and Axis"=w709, "Microstep Size (0)"=w708, "VISA resource name"=w712) -> ("error out"=w702:errorcluster)  [unwired: 3 in, 1 out]
            n461 = local write "ZaberError"(w702) -> ()
          }
          frame #2 {
            n462 = Tick Count (ms)() -> (millisecond timer value=w720:u32)
            n463 = Subtract(x=w720, y=w719) -> (x-y=w718:u32)
          }
          frame #3 {
            n464 = local read "Acc time [s]"() -> (w723:dbl)
            n465 = Multiply(x=1000.0 ("y"), y=w723) -> (x*y=w722:dbl)
            n466 = Add(x="AcqStartDelay", y=w722) -> (x+y=w721:dbl)
            n467 = Wait (ms)(milliseconds to wait=w721) -> ()  [unwired: 1 out]
          }
          frame #4 {
            n468 = Tick Count (ms)() -> (millisecond timer value=w728:u32)
            n469 = Subtract(x=w728, y=w727) -> (x-y=w726:u32)
          }
          frame #5 {
            # "acquisition command + waiting till acquisition is done (subVI is suppose to stop after finish)"
            n470 = Multiply(x="PresetVal", y=10.0) -> (x*y=w730:dbl)
            n471 = local read "X steps"() -> (w736:i32)
            n472 = local read "identifier out"() -> (w737:string)
            n473 = call "DANTE acquire multiple.vi"("Number of boards in chain"=u8 1, "Map points"=w736, "Time per spectrum [ms]"=w730, "identifier out"=w737) -> ("Statistics"=w729:dbl[][], "spectra"=w734:u16[][], "adv stats"=w733:u64[][])  [unwired: 5 in]
          }
          frame #6 {
            n474 = Tick Count (ms)() -> (millisecond timer value=w738:u32)
            n475 = Subtract(x=w738, y=w740) -> (x-y=w739:u32)
          }
          frame #7 {
            # "waiting till movement is completed - decelleration"
            n476 = local read "Assignment"() -> (w745:cluster{"Microstep Size":dbl, "Device":string}[])
            n477 = Index Array(array=w745, index=0) -> (element=w746:cluster{"Microstep Size":dbl, "Device":string})
            n478 = local read "ZaberError"() -> (w742:errorcluster)
            n479 = local read "Port"() -> (w747:refnum<visa-resource-name>)
            n480 = Unbundle(w746) -> ("Device"=w743:string)  [unwired: 1 out]
            n481 = call "Poll Until Idle.vi"("error in (no error)"=w742, "Device and Axis"=w743, "VISA resource name"=w747) -> ("error out"=w741:errorcluster)  [unwired: 7 in, 1 out]
            n482 = local write "ZaberError"(w741) -> ()
          }
          frame #8 {
            n483 = Tick Count (ms)() -> (millisecond timer value=w750:u32)
            n484 = Subtract(x=w750, y=w749) -> (x-y=w748:u32)
          }
          frame #9 {
            # "saving data"
            n485 = local read "ROI End"() -> (w753:u32)
            n486 = local read "ROI Begin"() -> (w754:u32)
            n487 = call "Extract LineData.vi"("ROI End"=w753, "Input Data"=w758, "ROI Beg"=w754) -> ("ROI Data"=w756:u32[], "Sum spectra"=→"Sum spectra per line":u32[])  [unwired: 1 out]
            n488 = local read "ROI map"() -> (w757:u32[][])
            n489 = local read "Line #"() -> (w752:i32)
            n490 = Replace Array Subset(array=w757, new element=w756, index (col)=w752) -> (w755:u32[][])  [unwired: 1 in]
            n491 = local write "ROI map"(w755) -> ()
            "Spectra" <- w758
          }
          frame #10 {
            w765 = "Map_" ("string")
            w767 = ";"
            n492 = local read "Data folder path"() -> (w761:path)
            n493 = local read "Line #"() -> (w768:i32)
            n494 = Get Date/Time In Seconds() -> (seconds since 1Jan1904=w771:timestamp)
            n495 = call "csv_names.vi"("Numeric"=w768) -> ("concatenated string"=w766:string)  [unwired: 1 in]
            n496 = Format Date/Time String(time format string (%c)="%04Y_%02m_%02d_%02H_%02M_%02S_", seconds (now)=w771, UTC format=FALSE ("want seconds? (F)")) -> (date/time string=w764:string)
            n497 = Concatenate Strings(w765, w764, w766, "_spectr.csv" ("string")) -> (w778:string)
            n498 = Concatenate Strings(w765, w764, w766, "_stats.csv" ("string")) -> (w762:string)
            n499 = Concatenate Strings(w765, w764, w766, "_advstat.csv" ("string")) -> (w773:string)
            n500 = Build Path(base path=w761, name or relative path=w778) -> (appended path=w777:path)
            n501 = Build Path(base path=w761, name or relative path=w773) -> (appended path=w772:path)
            n502 = Build Path(base path=w761, name or relative path=w762) -> (appended path=w760:path)
            n503 = call-poly <vilib>:"Write Delimited Spreadsheet.vi"("file path (dialog if empty)"=w777, "2D data"=w776, "delimiter (\\t)"=w767) -> ()  [unwired: 11 in, 2 out]
            n504 = call-poly <vilib>:"Write Delimited Spreadsheet.vi"("file path (dialog if empty)"=w772, "2D data"=w774, "delimiter (\\t)"=w767) -> ()  [unwired: 11 in, 2 out]
            n505 = call-poly <vilib>:"Write Delimited Spreadsheet.vi"("file path (dialog if empty)"=w760, "2D data"=w759, "delimiter (\\t)"=w767) -> ()  [unwired: 11 in, 2 out]
          }
          frame #11 {
            n506 = local read "total line #"() -> (w788:i32)
            n507 = local read "Line #"() -> (w781:i32)
            n508 = local read "scan timing [ms]"() -> (w782:dbl[][])
            n509 = Equal?(x=w788, y=w781) -> (x = y?=w789:bool)
            n510 = case shown="False" w789 {
              frame False {
                n511 = local read "Line #"() -> (w790:i32)
                n512 = Increment(x=w790) -> (x+1=w791:i32)
                n513 = local write "Line #"(w791) -> ()
              }
              frame True {
                n514 = local write "scan mode"(FALSE ("scan mode")) -> ()
              }
            }
            n515 = Build Array(w787, w786, w785, w784) -> (w783:u32[])
            n516 = Insert Into Array(array=w782, index (row)=w781, new element=w783) -> (w780:dbl[][])  [unwired: 1 in]
            n517 = local write "scan timing [ms]"(w780) -> ()
          }
        }
      }
      frame "Close" {
        n518 = local read "ZaberError"() -> (w796:errorcluster)
        n519 = local read "Port"() -> (w795:refnum<visa-resource-name>)
        n520 = call "Close.vi"("error in (no error)"=w796, "VISA resource name"=w795) -> ("error out"=→"ZaberError":errorcluster)  [unwired: 9 in]
      }
    }
    n521 = Wait Until Next ms Multiple(millisecond multiple=u32 1) -> ()  [unwired: 1 out]
    "Enum" <- w8
  }
